vi "(SubVI)Waveform Editor.vi"() -> ()   [LabVIEW 2020]
uses:
  Libraries/Waveform Obj Class/Waveform Gen/Controls/repeat scale.ctl
  Libraries/Waveform Obj Class/Square Wave/Controls/Slope Type.ctl
  Libraries/Waveform Obj Class/Waveform Obj/Waveform Obj.lvclass
  Controls/(Ctrl)Waveform Editor_Update Listbox User Event.ctl
  Controls/(Ctrl)Waveform Editor_WF List.ctl
  Controls/(Ctrl)Waveform Editor_Update Graph User Event.ctl
  <vilib>/Utility/miscctls.llb/LVPointTypeDef.ctl
  Mode Event/Controls/(Ctrl)Mode Event_FGV Function.ctl
  Controls/(Ctrl)Waveform Editor_Update Sampling Rate Value.ctl
  Libraries/Haptic IC Class/Haptic IC/Haptic IC.lvclass/Haptic IC.ctl
  Libraries/Waveform Obj Class/Waveform Gen/Controls/waveform gen type.ctl
  Libraries/Waveform Obj Class/Sine Wave/Sine Wave.lvclass
  Libraries/Waveform Obj Class/Square Wave/Square Wave.lvclass
  Libraries/Waveform Obj Class/Square Wave/Square Wave.lvclass/Square Wave.ctl
  Libraries/Waveform Obj Class/Triangle Wave/Triangle Wave.lvclass
  Libraries/Waveform Obj Class/Sawtooth Wave/Sawtooth Wave.lvclass
  Libraries/Waveform Obj Class/Auto Track Wave/Auto Track Wave.lvclass
  Libraries/Waveform Obj Class/Auto Brake (Square) Wave/Auto Brake (Square) Wave.lvclass
  Libraries/Waveform Obj Class/Auto Brake (Sine) Wave/Auto Brake (Sine) Wave.lvclass
  Libraries/Waveform Obj Class/PWL_DW7802/PWL_DW7802.lvclass
  Libraries/Waveform Obj Class/Waveform Gen/Waveform Gen.lvclass/Waveform Gen.ctl
  Libraries/Waveform Obj Class/Waveform Obj/Waveform Obj.lvclass/Waveform Obj.ctl
  Libraries/Waveform Obj Class/Waveform Gen/Waveform Gen.lvclass
  Libraries/Waveform Obj Class/PWL/PWL.lvclass
  Libraries/Waveform Obj Class/PWL/PWL.lvclass/PWL.ctl
  Libraries/Waveform Obj Class/WAV File/WAV File.lvclass
  Libraries/Waveform Obj Class/Text File/Text File.lvclass
  Libraries/Haptic IC Class/Haptic IC/Controls/(Ctrl)Mode.ctl
  Mode Event/Controls/(Ctrl)Mode Event_Event Type.ctl
  Libraries/Waveform Obj Class/Square Wave/Accessors/Write slope length.vi
  Libraries/Waveform Obj Class/Square Wave/Accessors/Write slope type.vi
  Libraries/Waveform Obj Class/Waveform Gen/Accessors/Write frequency.vi
  Libraries/Waveform Obj Class/Waveform Gen/Accessors/Write scale.vi
  Libraries/Waveform Obj Class/Waveform Gen/Accessors/Write cycle.vi
  Libraries/Waveform Obj Class/Waveform Gen/Accessors/Write repeat type.vi
  Libraries/Waveform Obj Class/Waveform Obj/Accessors/Write sampling rate.vi
  Libraries/Waveform Obj Class/Waveform Obj/Accessors/Write voltage range.vi
  Libraries/Waveform Obj Class/Waveform Obj/Accessors/Write wait.vi
  9968c254-cfa1-4b75-a9b0-3c7b6300c374.vi
  Libraries/Waveform Obj Class/Waveform Obj/Accessors/Write name.vi
  Libraries/Waveform Obj Class/Square Wave/Accessors/Read slope length.vi
  Libraries/Waveform Obj Class/Square Wave/Accessors/Read slope type.vi
  Libraries/Waveform Obj Class/PWL/Accessors/Read previous pwl scale.vi
  Libraries/Waveform Obj Class/PWL/Accessors/Read waveform type.vi
  Libraries/Waveform Obj Class/Waveform Gen/Accessors/Read frequency.vi
  Libraries/Waveform Obj Class/Waveform Gen/Accessors/Read scale.vi
  Libraries/Waveform Obj Class/Waveform Gen/Accessors/Read cycle.vi
  Libraries/Waveform Obj Class/Waveform Gen/Accessors/Read repeat type.vi
  Libraries/Waveform Obj Class/Waveform Obj/Accessors/Read play mode.vi
  Libraries/Waveform Obj Class/PWL/Accessors/Write waveform type.vi
  Libraries/Waveform Obj Class/Waveform Obj/Accessors/Write play mode.vi
  Libraries/Waveform Obj Class/PWL/Accessors/Write previous pwl scale.vi
  073afacf-4daa-4c2b-8e37-4aa6efe5eb82.vi
  Libraries/Waveform Obj Class/Waveform Obj/Accessors/Read name.vi
  Libraries/Waveform Obj Class/Waveform Obj/Accessors/Read wait.vi
  Variables/(Var)System Variables.vi
  <vilib>/Comparison/Less/Less Functor/Less Functor.lvclass
  Libraries/Haptic IC Class/Haptic IC/Haptic IC.lvclass
panel:
  in  "WF Seq_PWL Points":u8(ring)=1 caption="PWL points" items=["1"=1, "2"=2, "3"=3, "4"=4, "5"=5, "6"=6, "7"=7]
  in  "WF Seq_Play Mode":u8(ring)
  in  "WF Seq_PWL_DW7802":T1(array[cluster])=[{"Shape"=0, "Ramp"=0, "Amplitude"=1.0, "Frequency"=100.0, "Cycle"=1.0}] {"Frequency" min=40.0 max=300.0 step=1.0; "Cycle" items=["0.5"=0.5, "1"=1.0, "1.5"=1.5, "2"=2.0, "2.5"=2.5, "3"=3.0, "3.5"=3.5, "4"=4.0, "4.5"=4.5, "5"=5.0, "5.5"=5.5, "6"=6.0, "6.5"=6.5, "7"=7.0, "7.5"=7.5, "8"=8.0, "8.5"=8.5, "9"=9.0, "9.5"=9.5, "10"=10.0, "10.5"=10.5, "11"=11.0, "11.5"=11.5, "12"=12.0, "12.5"=12.5, "13"=13.0, "13.5"=13.5, "14"=14.0, "14.5"=14.5, "15"=15.0, "15.5"=15.5, "16"=16.0, "16.5"=16.5, "17"=17.0, "17.5"=17.5, "18"=18.0, "18.5"=18.5, "19"=19.0, "19.5"=19.5, "20"=20.0, "20.5"=20.5, "21"=21.0, "21.5"=21.5, "22"=22.0, "22.5"=22.5, "23"=23.0, "23.5"=23.5, "24"=24.0, "24.5"=24.5, "25"=25.0, "25.5"=25.5, "26"=26.0, "26.5"=26.5, "27"=27.0, "27.5"=27.5, "28"=28.0, "28.5"=28.5, "29"=29.0, "29.5"=29.5, "30"=30.0, "30.5"=30.5, "31"=31.0, "31.5"=31.5, "32"=32.0, "32.5"=32.5, "33"=33.0, "33.5"=33.5, "34"=34.0, "34.5"=34.5, "35"=35.0, "35.5"=35.5, "36"=36.0, "36.5"=36.5, "37"=37.0, "37.5"=37.5, "38"=38.0, "38.5"=38.5, "39"=39.0, "39.5"=39.5, "40"=40.0, "40.5"=40.5, "41"=41.0, "41.5"=41.5, "42"=42.0, "42.5"=42.5, "43"=43.0, "43.5"=43.5, "44"=44.0, "44.5"=44.5, "45"=45.0, "45.5"=45.5, "46"=46.0, "46.5"=46.5, "47"=47.0, "47.5"=47.5, "48"=48.0, "48.5"=48.5, "49"=49.0, "49.5"=49.5, "50"=50.0, "50.5"=50.5, "51"=51.0, "51.5"=51.5, "52"=52.0, "52.5"=52.5, "53"=53.0, "53.5"=53.5, "54"=54.0, "54.5"=54.5, "55"=55.0, "55.5"=55.5, "56"=56.0, "56.5"=56.5, "57"=57.0, "57.5"=57.5, "58"=58.0, "58.5"=58.5, "59"=59.0, "59.5"=59.5, "60"=60.0, "60.5"=60.5, "61"=61.0, "61.5"=61.5, "62"=62.0, "62.5"=62.5, "63"=63.0, "63.5"=63.5, "64"=64.0, "64.5"=64.5, "65"=65.0, "65.5"=65.5, "66"=66.0, "66.5"=66.5, "67"=67.0, "67.5"=67.5, "68"=68.0, "68.5"=68.5, "69"=69.0, "69.5"=69.5, "70"=70.0, "70.5"=70.5, "71"=71.0, "71.5"=71.5, "72"=72.0, "72.5"=72.5, "73"=73.0, "73.5"=73.5, "74"=74.0, "74.5"=74.5, "75"=75.0, "75.5"=75.5, "76"=76.0, "76.5"=76.5, "77"=77.0, "77.5"=77.5, "78"=78.0, "78.5"=78.5, "79"=79.0, "79.5"=79.5, "80"=80.0, "80.5"=80.5, "81"=81.0, "81.5"=81.5, "82"=82.0, "82.5"=82.5, "83"=83.0, "83.5"=83.5, "84"=84.0, "84.5"=84.5, "85"=85.0, "85.5"=85.5, "86"=86.0, "86.5"=86.5, "87"=87.0, "87.5"=87.5, "88"=88.0, "88.5"=88.5, "89"=89.0, "89.5"=89.5, "90"=90.0, "90.5"=90.5, "91"=91.0, "91.5"=91.5, "92"=92.0, "92.5"=92.5, "93"=93.0, "93.5"=93.5, "94"=94.0, "94.5"=94.5, "95"=95.0, "95.5"=95.5, "96"=96.0, "96.5"=96.5, "97"=97.0, "97.5"=97.5, "98"=98.0, "98.5"=98.5, "99"=99.0, "99.5"=99.5, "100"=100.0, "100.5"=100.5, "101"=101.0, "101.5"=101.5, "102"=102.0, "102.5"=102.5, "103"=103.0, "103.5"=103.5, "104"=104.0, "104.5"=104.5, "105"=105.0, "105.5"=105.5, "106"=106.0, "106.5"=106.5, "107"=107.0, "107.5"=107.5, "108"=108.0, "108.5"=108.5, "109"=109.0, "109.5"=109.5, "110"=110.0, "110.5"=110.5, "111"=111.0, "111.5"=111.5, "112"=112.0, "112.5"=112.5, "113"=113.0, "113.5"=113.5, "114"=114.0, "114.5"=114.5, "115"=115.0, "115.5"=115.5, "116"=116.0, "116.5"=116.5, "117"=117.0, "117.5"=117.5, "118"=118.0, "118.5"=118.5, "119"=119.0, "119.5"=119.5, "120"=120.0, "120.5"=120.5, "121"=121.0, "121.5"=121.5, "122"=122.0, "122.5"=122.5, "123"=123.0, "123.5"=123.5, "124"=124.0, "124.5"=124.5, "125"=125.0, "125.5"=125.5, "126"=126.0, "126.5"=126.5, "127"=127.0, "127.5"=127.5]; "Amplitude" items=["0"=0.0, "10"=0.1, "20"=0.2, "30"=0.3, "40"=0.4, "50"=0.5, "60"=0.6, "70"=0.7, "80"=0.8, "90"=0.9, "100"=1.0]; "Ramp" items=["Step"=0, "Ramp (Lin.)"=2, "Ramp (Exp.)"=3]; "Shape" items=["Sine", "Square"]}
  in  "WF Seq_PWL Listbox":i32[](listbox)
  out "WF Gen_Auto Tracking Waring":string="Warning!\nThe center frequency of tracking range is out of range in the default ZXD Setting."
  in  "WF Seq_Wait":u8(ring) caption="Wait" items=["0us", "166us", "332us", "498us", "664us", "830us", "996us", "1162us", "1328us", "1494us", "1660us", "1826us", "1992us", "2158us", "2324us", "2490us"]
  in  "WF List_Mem Update":bool
  in  "WF List_RTP Stop":bool
  in  "WF List_RTP Start":bool
  in  "WF Seq_Voltage Range":dbl(ring) caption="VD Clamp" items=["0.00V"=0.0, "0.04V"=0.04, "0.08V"=0.08, "0.12V"=0.12, "0.16V"=0.16, "0.20V"=0.2, "0.24V"=0.24, "0.28V"=0.28, "0.32V"=0.32, "0.36V"=0.36, "0.40V"=0.4, "0.44V"=0.44, "0.48V"=0.48, "0.52V"=0.52, "0.56V"=0.56, "0.60V"=0.6, "0.64V"=0.64, "0.68V"=0.68, "0.72V"=0.72, "0.76V"=0.76, "0.80V"=0.8, "0.84V"=0.84, "0.88V"=0.88, "0.92V"=0.92, "0.96V"=0.96, "1.00V"=1.0, "1.04V"=1.04, "1.08V"=1.08, "1.12V"=1.12, "1.16V"=1.16, "1.20V"=1.2, "1.24V"=1.24, "1.28V"=1.28, "1.32V"=1.32, "1.36V"=1.36, "1.40V"=1.4, "1.44V"=1.44, "1.48V"=1.48, "1.52V"=1.52, "1.56V"=1.56, "1.60V"=1.6, "1.64V"=1.64, "1.68V"=1.68, "1.72V"=1.72, "1.76V"=1.76, "1.80V"=1.8, "1.84V"=1.84, "1.88V"=1.88, "1.92V"=1.92, "1.96V"=1.96, "2.00V"=2.0, "2.04V"=2.04, "2.08V"=2.08, "2.12V"=2.12, "2.16V"=2.16, "2.20V"=2.2, "2.24V"=2.24, "2.28V"=2.28, "2.32V"=2.32, "2.36V"=2.36, "2.40V"=2.4, "2.44V"=2.44, "2.48V"=2.48, "2.52V"=2.52, "2.56V"=2.56, "2.60V"=2.6, "2.64V"=2.64, "2.68V"=2.68, "2.72V"=2.72, "2.76V"=2.76, "2.80V"=2.8, "2.84V"=2.84, "2.88V"=2.88, "2.92V"=2.92, "2.96V"=2.96, "3.00V"=3.0, "3.04V"=3.04, "3.08V"=3.08, "3.12V"=3.12, "3.16V"=3.16, "3.20V"=3.2, "3.24V"=3.24, "3.28V"=3.28, "3.32V"=3.32, "3.36V"=3.36, "3.40V"=3.4, "3.44V"=3.44, "3.48V"=3.48, "3.52V"=3.52, "3.56V"=3.56, "3.60V"=3.6, "3.64V"=3.64, "3.68V"=3.68, "3.72V"=3.72, "3.76V"=3.76, "3.80V"=3.8, "3.84V"=3.84, "3.88V"=3.88, "3.92V"=3.92, "3.96V"=3.96, "4.00V"=4.0, "4.04V"=4.04, "4.08V"=4.08, "4.12V"=4.12, "4.16V"=4.16, "4.20V"=4.2, "4.24V"=4.24, "4.28V"=4.28, "4.32V"=4.32, "4.36V"=4.36, "4.40V"=4.4, "4.44V"=4.44, "4.48V"=4.48, "4.52V"=4.52, "4.56V"=4.56, "4.60V"=4.6, "4.64V"=4.64, "4.68V"=4.68, "4.72V"=4.72, "4.76V"=4.76, "4.80V"=4.8, "4.84V"=4.84, "4.88V"=4.88, "4.92V"=4.92, "4.96V"=4.96, "5.00V"=5.0, "5.04V"=5.04, "5.08V"=5.08, "5.12V"=5.12, "5.16V"=5.16, "5.20V"=5.2, "5.24V"=5.24, "5.28V"=5.28, "5.32V"=5.32, "5.36V"=5.36, "5.40V"=5.4, "5.44V"=5.44, "5.48V"=5.48, "5.52V"=5.52, "5.56V"=5.56, "5.60V"=5.6, "5.64V"=5.64, "5.68V"=5.68, "5.72V"=5.72, "5.76V"=5.76, "5.80V"=5.8, "5.84V"=5.84, "5.88V"=5.88, "5.92V"=5.92, "5.96V"=5.96, "6.00V"=6.0, "6.04V"=6.04, "6.08V"=6.08, "6.12V"=6.12, "6.16V"=6.16, "6.20V"=6.2, "6.24V"=6.24, "6.28V"=6.28, "6.32V"=6.32, "6.36V"=6.36, "6.40V"=6.4, "6.44V"=6.44, "6.48V"=6.48, "6.52V"=6.52, "6.56V"=6.56, "6.60V"=6.6, "6.64V"=6.64, "6.68V"=6.68, "6.72V"=6.72, "6.76V"=6.76, "6.80V"=6.8, "6.84V"=6.84, "6.88V"=6.88, "6.92V"=6.92, "6.96V"=6.96, "7.00V"=7.0, "7.04V"=7.04, "7.08V"=7.08, "7.12V"=7.12, "7.16V"=7.16, "7.20V"=7.2, "7.24V"=7.24, "7.28V"=7.28, "7.32V"=7.32, "7.36V"=7.36, "7.40V"=7.4, "7.44V"=7.44, "7.48V"=7.48, "7.52V"=7.52, "7.56V"=7.56, "7.60V"=7.6, "7.64V"=7.64, "7.68V"=7.68, "7.72V"=7.72, "7.76V"=7.76, "7.80V"=7.8, "7.84V"=7.84, "7.88V"=7.88, "7.92V"=7.92, "7.96V"=7.96, "8.00V"=8.0, "8.04V"=8.04, "8.08V"=8.08, "8.12V"=8.12, "8.16V"=8.16, "8.20V"=8.2, "8.24V"=8.24, "8.28V"=8.28, "8.32V"=8.32, "8.36V"=8.36, "8.40V"=8.4, "8.44V"=8.44, "8.48V"=8.48, "8.52V"=8.52, "8.56V"=8.56, "8.60V"=8.6, "8.64V"=8.64, "8.68V"=8.68, "8.72V"=8.72, "8.76V"=8.76, "8.80V"=8.8, "8.84V"=8.84, "8.88V"=8.88, "8.92V"=8.92, "8.96V"=8.96, "9.00V"=9.0, "9.04V"=9.04, "9.08V"=9.08, "9.12V"=9.12, "9.16V"=9.16, "9.20V"=9.2, "9.24V"=9.24, "9.28V"=9.28, "9.32V"=9.32, "9.36V"=9.36, "9.40V"=9.4, "9.44V"=9.44, "9.48V"=9.48, "9.52V"=9.52, "9.56V"=9.56, "9.60V"=9.6, "9.64V"=9.64, "9.68V"=9.68, "9.72V"=9.72, "9.76V"=9.76, "9.80V"=9.8, "9.84V"=9.84, "9.88V"=9.88, "9.92V"=9.92, "9.96V"=9.96, "10.00V"=10.0, "10.04V"=10.04, "10.08V"=10.08, "10.12V"=10.12, "10.16V"=10.16, "10.20V"=10.2]
  in  "WF List_Import":bool
  out "Graph_Cursor Y":dbl caption="Y :" format="Y : %#.3f"
  out "Graph_Cursor X":dbl caption="Cursor X :" format="X : %#_g"
  out "WF List_Total Bytes":i32 caption="Total :" format="%d Byte"
  out "WF Seq_Total Bytes":i32 caption="Total :" format="%d Byte"
  out "Graph":dbl[](graph)
  in  "WF List_Export":bool
  in  "WF List_Load File":bool
  in  "WF List_Save File":bool
  in  "WF List_Delete":bool
  in  "WF List_Rename":bool
  in  "WF List_Down":bool
  in  "WF List_Up":bool
  in  "WF List_View":bool
  in  "WF Seq_Change":bool
  in  "WF Seq_Add to List":bool
  in  "WF Seq_Load File":bool
  in  "WF Seq_Save File":bool
  in  "WF Seq_Delete":bool
  in  "WF Seq_Rename":bool
  in  "WF Seq_Down":bool
  in  "WF Seq_Up":bool
  in  "WF Seq_View":bool
  in  "WF Gen_Change":bool
  in  "WF Gen_Add to Seq":bool
  in  "WF List_Sampling Rate":u32(ring)=8000 caption="PWM" items=["24kHz"=24000, "48kHz"=48000, "96kHz"=96000, "12kHz"=12000]
  in  "WF Seq":i32[](listbox)
  in  "WF List":i32[](listbox)
  in  "WF Gen_Setting":T4={"Waveform Type"=0, "Freq."=160.0, "Scale"=1.0, "Cycle"=1.0, "Repeat Type"=enum."Normal", "Square_Slope Length"=25, "Square_Slope"=enum."Exp."} {"Scale" min=-1.0 max=1.0; "Waveform Type" items=["Sine", "Square", "Triangle", "Sawtooth"]}
  # "Waveform Editor"
  # "Cursor"
  # "Waveform Generate"
  # "Waveform Build"
  # "Waveform List"
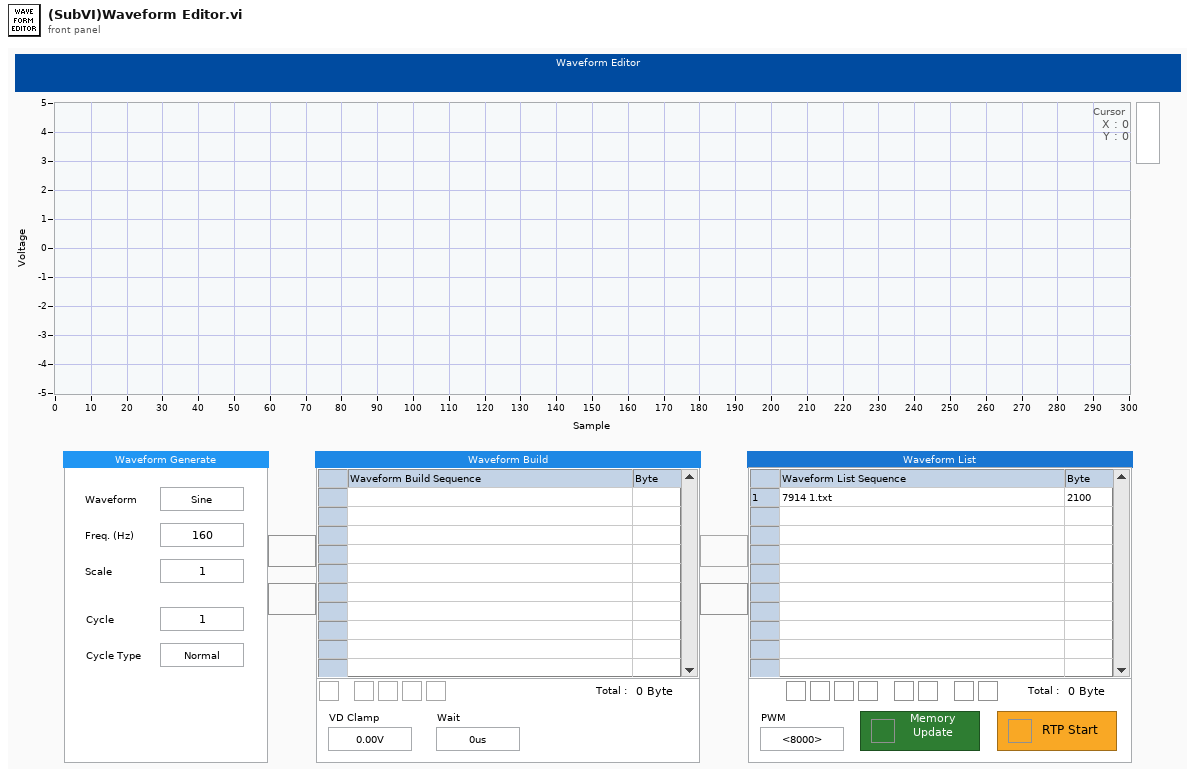
[diagram p1: front panel]
types:
  T1 = cluster{"Shape":u16, "Ramp":u16, "Amplitude":dbl, "Frequency":dbl, "Cycle":dbl}[]
  T2 = typedef "Waveform Gen.lvclass/repeat scale.ctl" = enum16{"Normal", "Lin. Up", "Lin. Down", "Exp. Up", "Exp. Down"}
  T3 = typedef "Square Wave.lvclass/Slope Type.ctl" = enum16{"None", "Lin.", "Exp."}
  T4 = cluster{"Waveform Type":u16, "Freq.":dbl, "Scale":dbl, "Cycle":dbl, "Repeat Type":T2, "Square_Slope Length":u32, "Square_Slope":T3}
  T5 = typedef "(Ctrl)Mode Event_FGV Function.ctl" = enum16{"Init", "Get Event Ref", "Gen Event", "Destroy"}
  T6 = typedef "LVPointTypeDef.ctl" = cluster{"Horizontal":i16, "Vertical":i16}
  T7 = typedef "(Ctrl)Waveform Editor_Update Graph User Event.ctl" = enum16{"WF Gen", "WF Seq", "Latest"}
  T8 = typedef "(Ctrl)Waveform Editor_Update Listbox User Event.ctl" = enum16{"WF Seq", "WF List"}
  T9 = typedef "(Ctrl)Waveform Editor_WF List.ctl" = cluster{"Name":string, "WF Seq":refnum<class "Waveform Obj.lvclass">[]}
  T10 = typedef "(Ctrl)Waveform Editor_Update Sampling Rate Value.ctl" = enum16{"Init", "Update"}
  T11 = typedef "Haptic IC.lvclass/(Ctrl)IC Type.ctl" = enum8{"DW7800", "DW7802", "DW7912", "DW7914"}
  T12 = typedef "Waveform Gen.lvclass/waveform gen type.ctl" = enum16{"Sine", "Square", "Triangle", "Sawtooth", "Auto Track", "Auto Brake (Square)", "Auto Brake (Sine)", "PWL"}
  T13 = typedef "LVStringsAndValuesArrayTypeDef_DBL.ctl" = cluster{"String":string, "Value":dbl}[]
  T14 = typedef "LVStringsAndValuesArrayTypeDef_U32.ctl" = cluster{"String":string, "Value":u32}[]
  T15 = typedef "LVStringsAndValuesArrayTypeDef_U8.ctl" = cluster{"String":string, "Value":u8}[]
  T16 = enum16{"open", "replace", "create", "open or create", "replace or create", "replace or create with confirmation"}
  T17 = enum8{"Enabled", "Disabled", "Disabled and Grayed Out"}
  T18 = typedef "(Ctrl)Waveform Editor_Update Graph User Event.ctl" = enum16{"WF Gen", "WF Seq", "WF List", "Latest"}
  T19 = typedef "(Ctrl)Mode.ctl" = enum16{"RTP", "Memory"}
  T20 = typedef "(Ctrl)Mode Event_Event Type.ctl" = enum16{"RTP Play", "RTP Stop", "Scope Start", "Scope Stop"}
  T21 = typedef "LVRowAndColumnTypeDef.ctl" = cluster{"Row":i32, "Column":i32}
  T22 = typedef "LVPoint32TypeDef.ctl" = cluster{"Horizontal":i32, "Vertical":i32}
  T23 = cluster{"Shape":u16, "Ramp":u16, "Amplitude":dbl, "Frequency":dbl, "Cycle":dbl}
  T24 = cluster{"Accessors:waveform type":T12, "Accessors:repeat type":T2, "Accessors:scale":dbl, "Accessors:frequency":dbl, "Accessors:cycle":dbl}
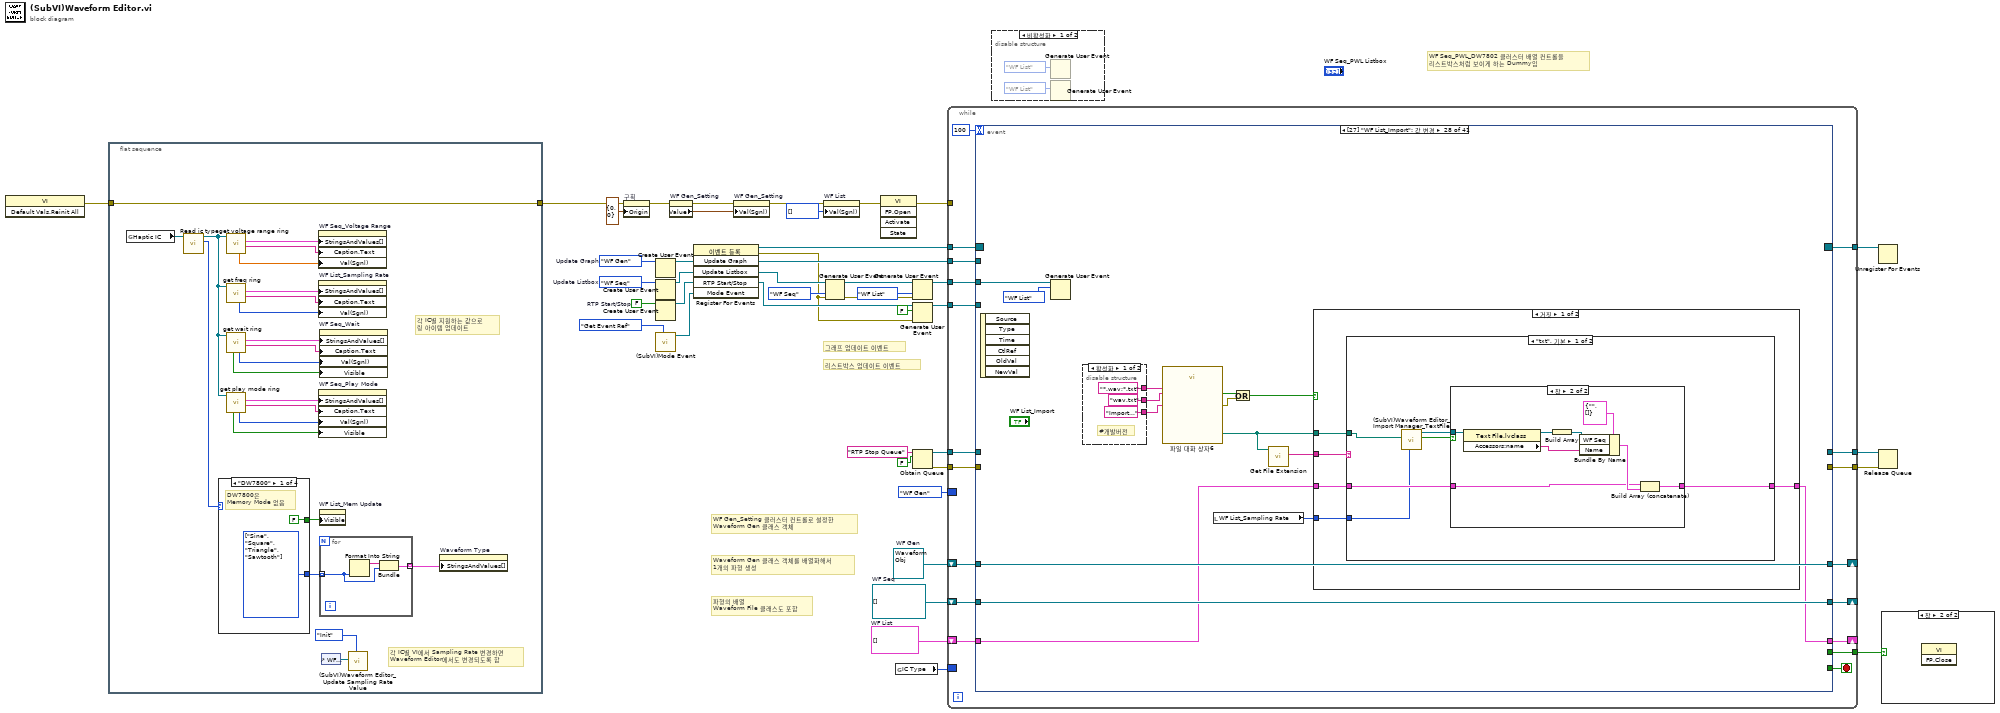
[diagram p0: block diagram]
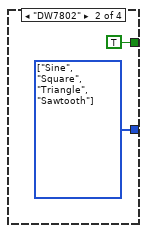
[diagram p3: hidden frame]
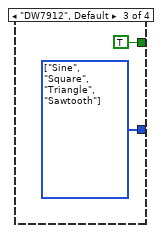
[diagram p4: hidden frame]
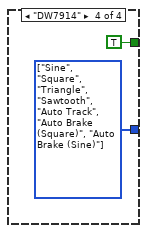
[diagram p5: hidden frame]
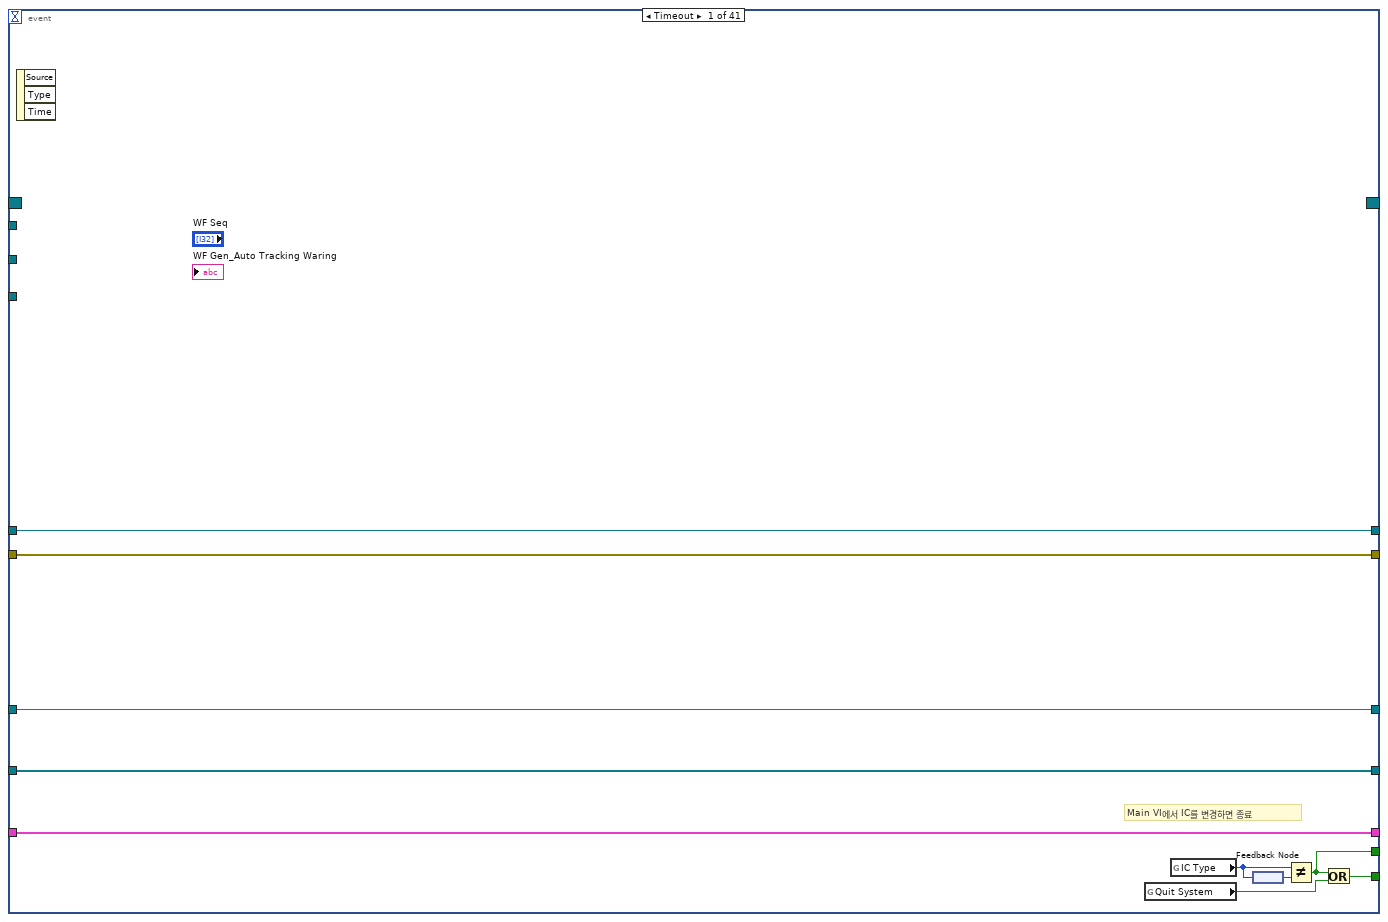
[diagram p7: hidden frame]
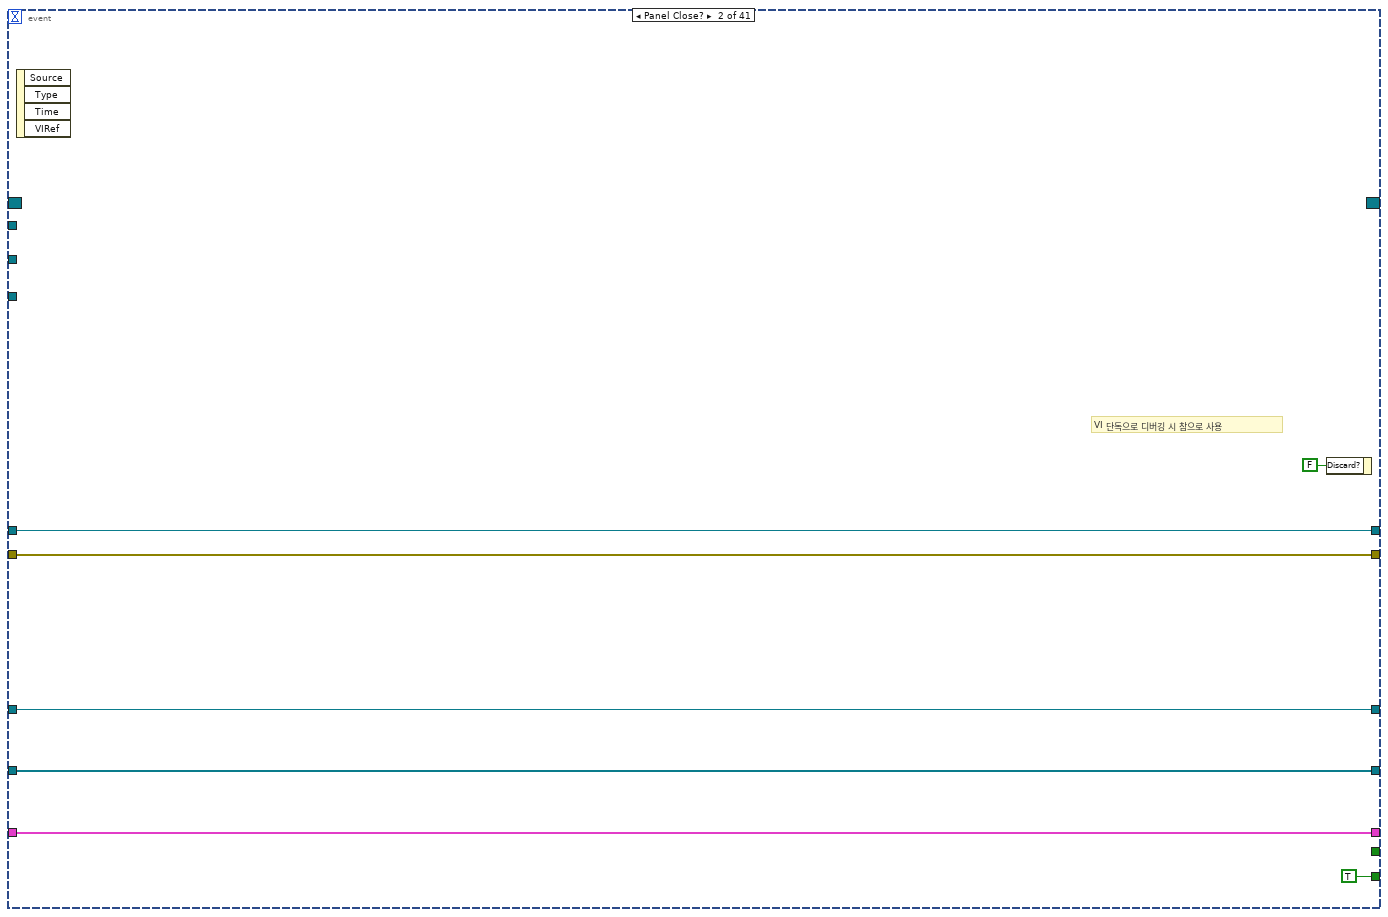
[diagram p8: hidden frame]
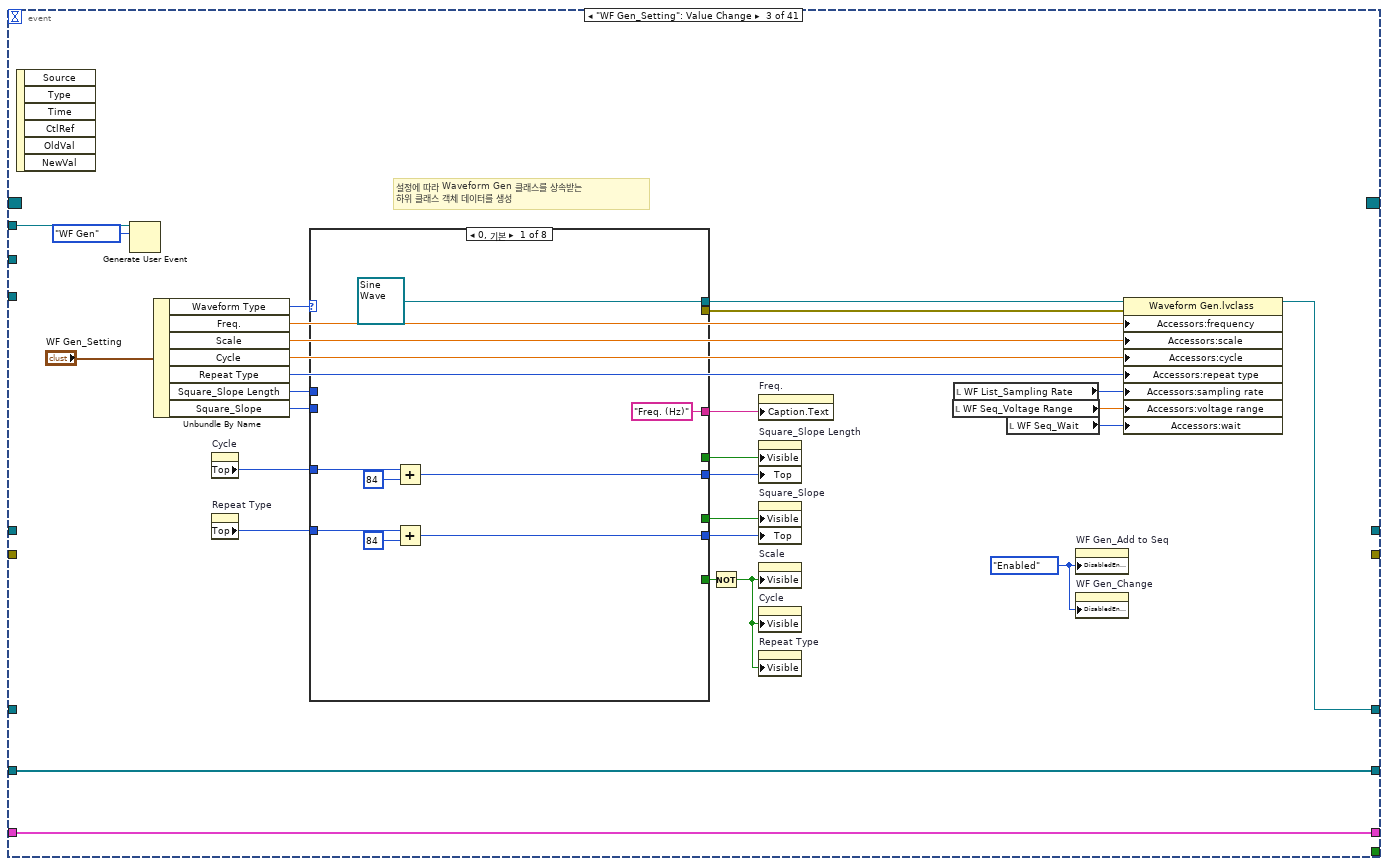
[diagram p9: hidden frame]
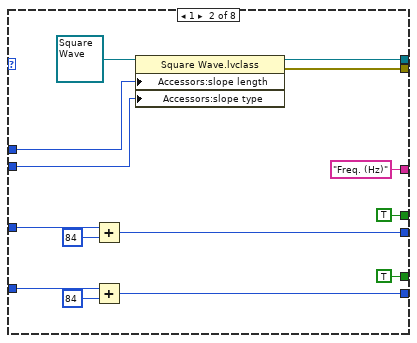
[diagram p10: hidden frame]
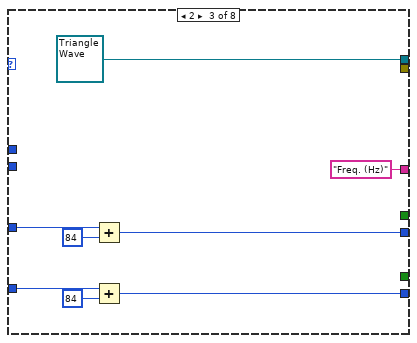
[diagram p11: hidden frame]
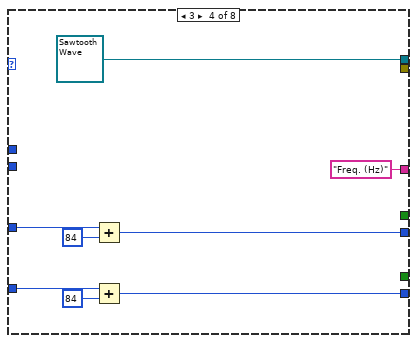
[diagram p12: hidden frame]
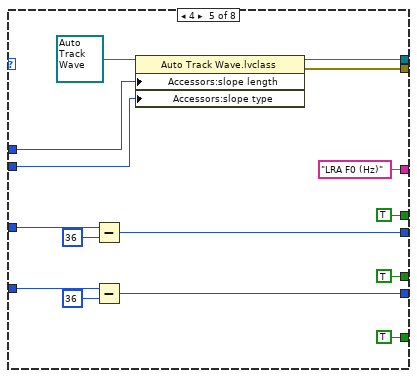
[diagram p13: hidden frame]
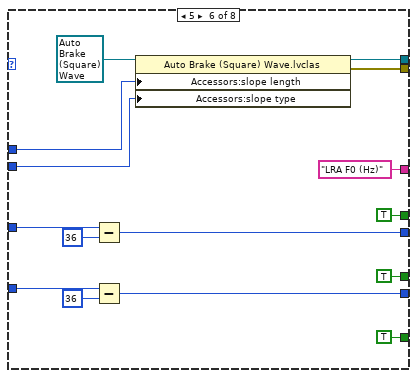
[diagram p14: hidden frame]
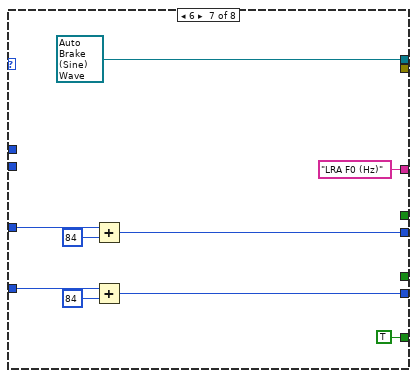
[diagram p15: hidden frame]
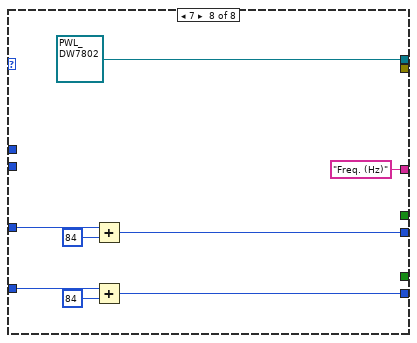
[diagram p16: hidden frame]
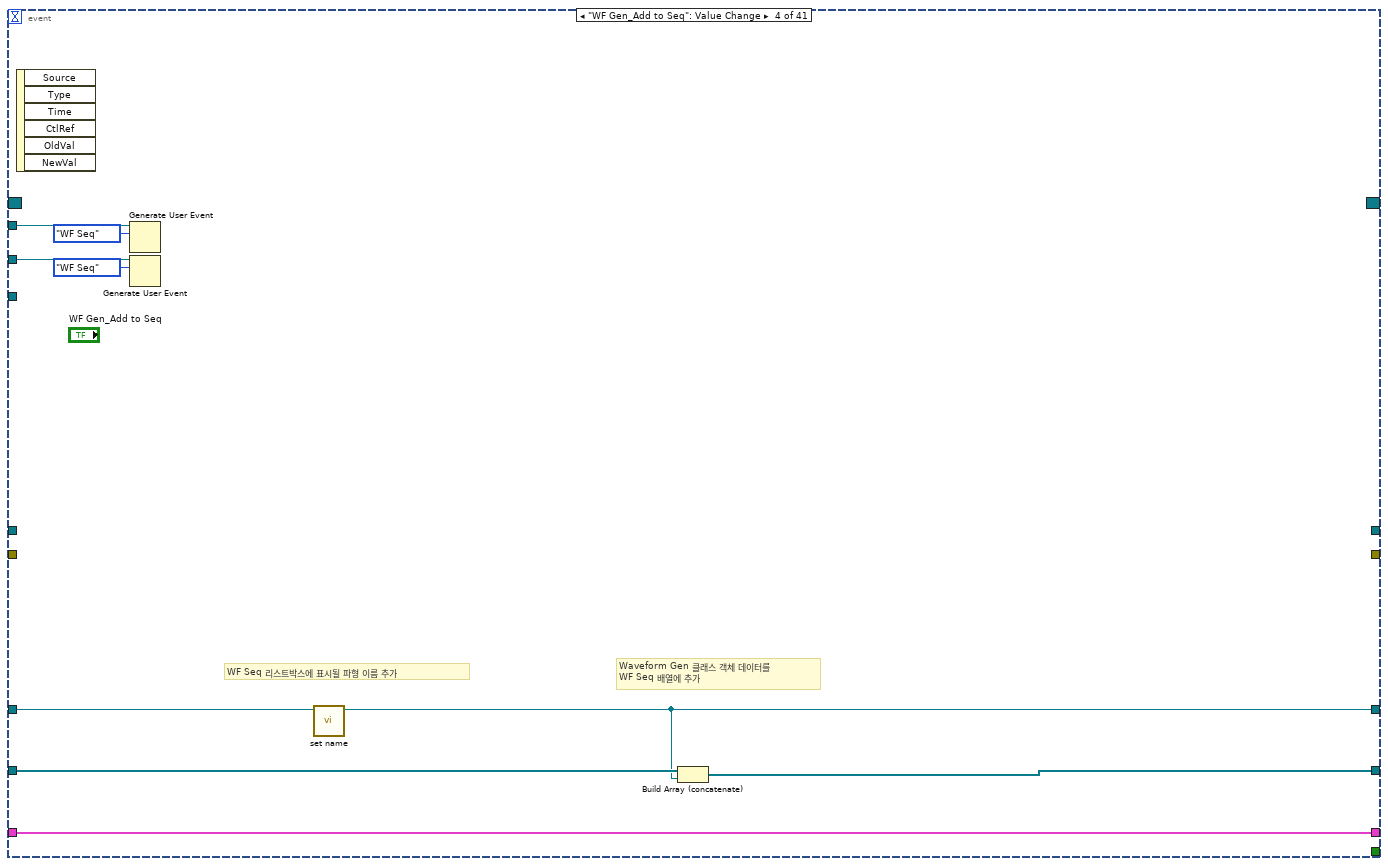
[diagram p17: hidden frame]
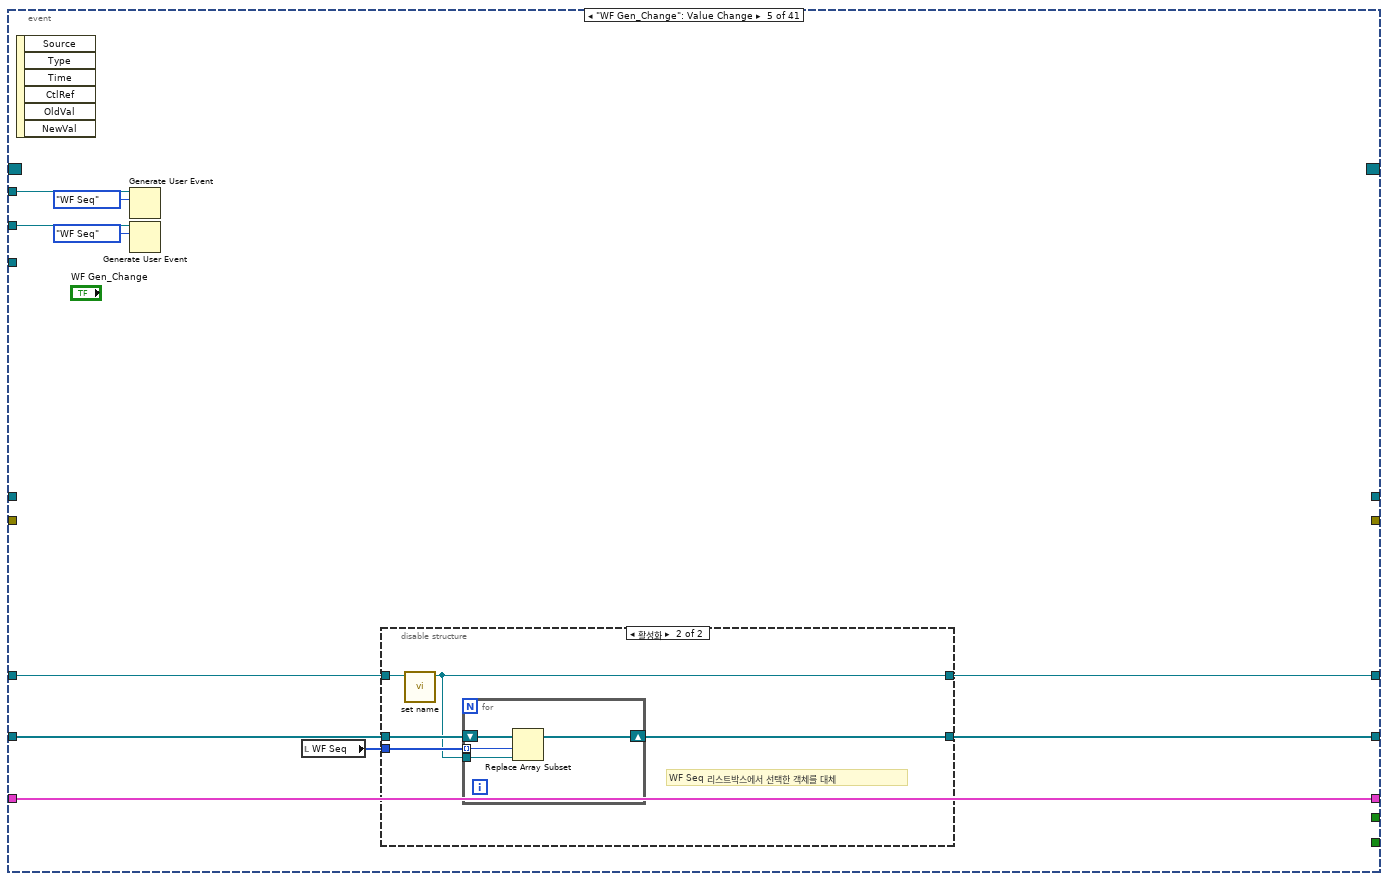
[diagram p18: hidden frame]
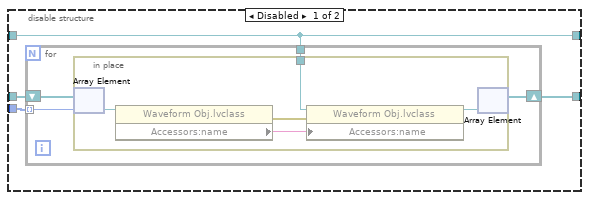
[diagram p19: hidden frame]
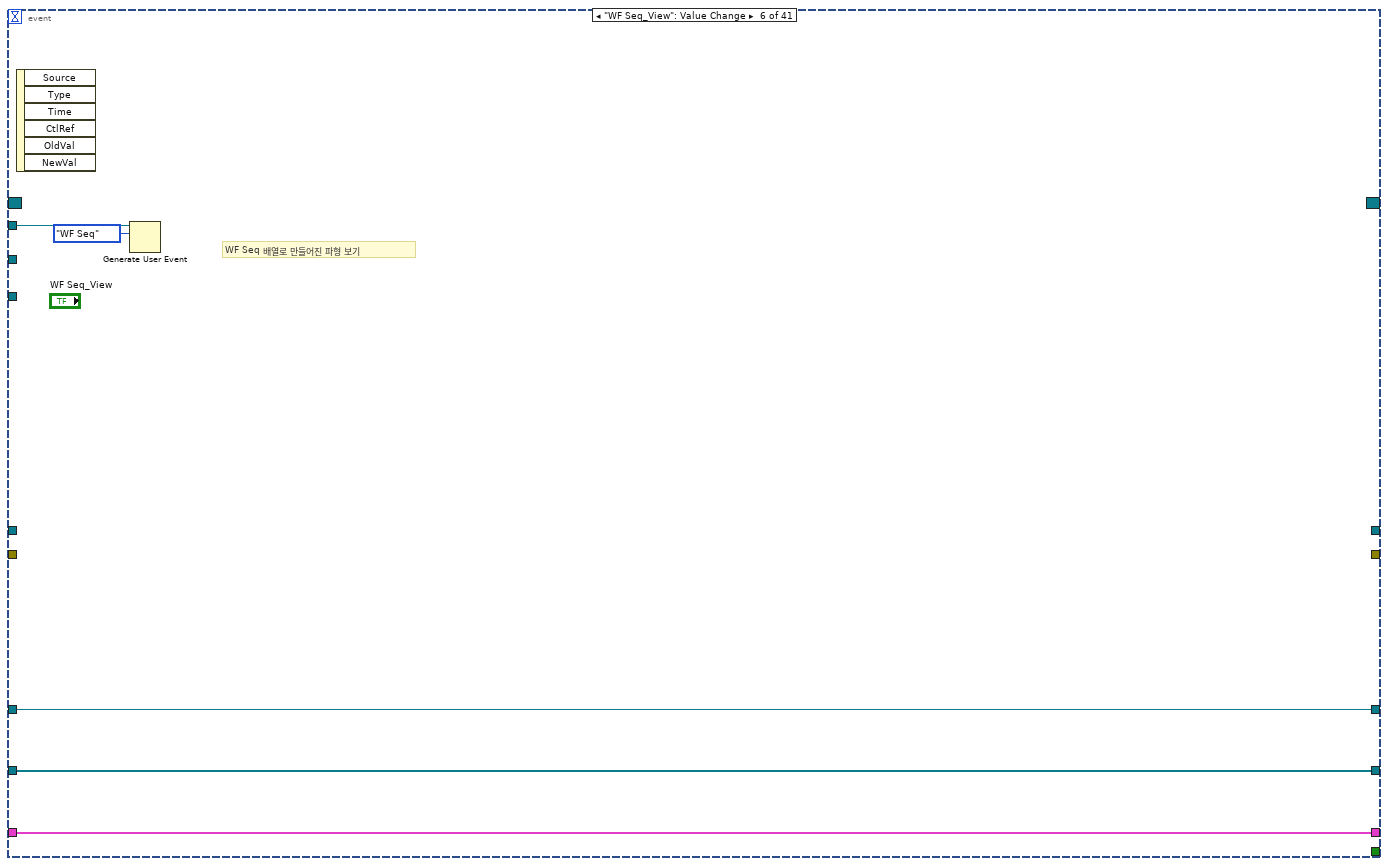
[diagram p20: hidden frame]
diagram:
  w14 = FALSE  # RTP Start/Stop
  w21 = T9[] []  # WF List
  w33 = (Ctrl)Waveform_Editor_Update_Listbox_User_Event."WF Seq"  # Update Listbox
  w36 = (Ctrl)Waveform_Editor_Update_Graph_User_Event."WF Gen"  # Update Graph
  w39 = refnum<class "Waveform Obj.lvclass"> refnum  # WF Gen
  w40 = refnum<class "Waveform Obj.lvclass">[] []  # WF Seq
  # "WF Seq_PWL_DW7802 클러스터 배열 컨트롤을\n리스트박스처럼 보이게 하는 Dummy임"
  # "리스트박스 업데이트 이벤트"
  # "그래프 업데이트 이벤트"
  # "파형의 배열\nWaveform File 클래스도 포함"
  # "Waveform Gen 클래스 객체를 배열화해서\n1개의 파형 생성"
  # "WF Gen_Setting 클러스터 컨트롤로 설정한\nWaveform Gen 클래스 객체"
  n1 = invoke class="VI" method="Default Vals.Reinit All"() -> (error out=w8:errorcluster)  [unwired: 3 in, 2 out]
  n2 = flat-sequence {
    tunnel: w8 -> [w56]
    tunnel: [w56] -> w6
    frame #0 {
      # "각 IC별 지원하는 값으로\n링 아이템 업데이트"
      # "각 IC별 VI에서 Sampling Rate 변경하면\nWaveform Editor에서도 변경되도록 함"
      n3 = global read "(Var)System Variables.vi" "Haptic IC"() -> (w59:refnum<class "Haptic IC.lvclass">)
      n4 = call "Read ic type.vi"("Haptic IC 입력"=w59) -> ("ic type"=w58:T11, "Haptic IC 출력"=w41:refnum<class "Haptic IC.lvclass">)  [unwired: 8 in, 1 out]
      n5 = case shown="\"DW7800\"" w58 {
        tunnel: [FALSE TRUE TRUE TRUE] -> w57
        tunnel: [w67 w69 w71 w73] -> w49
        frame "DW7800" {
          w67 = T12[] [enum."Sine", enum."Square", enum."Triangle", enum."Sawtooth"] items=["Sine", "Square", "Triangle", "Sawtooth", "Auto Track", "Auto Brake (Square)", "Auto Brake (Sine)", "PWL"] ("배열")
          # "DW7800은 \nMemory Mode 없음"
        }
        frame "DW7802" {
          w69 = T12[] [enum."Sine", enum."Square", enum."Triangle", enum."Sawtooth"] items=["Sine", "Square", "Triangle", "Sawtooth", "Auto Track", "Auto Brake (Square)", "Auto Brake (Sine)", "PWL"] ("배열")
        }
        frame "DW7912", Default {
          w71 = T12[] [enum."Sine", enum."Square", enum."Triangle", enum."Sawtooth"] items=["Sine", "Square", "Triangle", "Sawtooth", "Auto Track", "Auto Brake (Square)", "Auto Brake (Sine)", "PWL"] ("배열")
        }
        frame "DW7914" {
          w73 = T12[] [enum."Sine", enum."Square", enum."Triangle", enum."Sawtooth", enum."Auto Track", enum."Auto Brake (Square)", enum."Auto Brake (Sine)"] items=["Sine", "Square", "Triangle", "Sawtooth", "Auto Track", "Auto Brake (Square)", "Auto Brake (Sine)", "PWL"] ("배열")
        }
      }
      n6 = call-dynamic "get voltage range ring.vi"("Haptic IC 입력"=w41) -> ("caption"=w63:string, "strings & values"=w61:T13, "read value"=w51:dbl)  [unwired: 6 in, 2 out]
      n7 = call-dynamic "get freq ring.vi"("Haptic IC 입력"=w41) -> ("caption"=w62:string, "strings & values"=w60:T14, "read value"=w50:u32)  [unwired: 6 in, 2 out]
      n8 = call-dynamic "get wait ring.vi"("Haptic IC 입력"=w41) -> ("caption"=w54:string, "strings & values"=w55:T15, "default value"=w53:u8, "using"=w52:bool)  [unwired: 5 in, 2 out]
      n9 = call-dynamic "get play mode ring.vi"("Haptic IC 입력"=w41) -> ("caption"=w44:string, "strings & values"=w43:T15, "default value"=w45:u8, "using"=w42:bool)  [unwired: 5 in, 2 out]
      n10 = property on="WF Seq_Voltage Range" class="Ring (엄격한)"("StringsAndValues[]"=w61, "Caption.Text"=w63, "Val(Sgnl)"=w51) -> ()  [unwired: 2 in, 2 out]
      n11 = property on="WF List_Sampling Rate" class="Ring (엄격한)"("StringsAndValues[]"=w60, "Caption.Text"=w62, "Val(Sgnl)"=w50) -> ()  [unwired: 2 in, 2 out]
      n12 = property on="WF Seq_Play Mode" class="Ring (엄격한)"("StringsAndValues[]"=w43, "Caption.Text"=w44, "Val(Sgnl)"=w45, "Visible"=w42) -> ()  [unwired: 2 in, 2 out]
      n13 = property on="WF Seq_Wait" class="Ring (엄격한)"("StringsAndValues[]"=w55, "Caption.Text"=w54, "Val(Sgnl)"=w53, "Visible"=w52) -> ()  [unwired: 2 in, 2 out]
      n14 = property on="WF List_Mem Update" class="Bool"("Visible"=w57) -> ()  [unwired: 2 in, 2 out]
      n15 = for {
        tunnel: w49 -> [w65] mode=indexing
        tunnel: [w64] -> w48 mode=indexing
        n16 = Format Into String(w65) -> (resulting string=w66:string)  [unwired: 3 in, 1 out]
        n17 = Bundle(w66, "Waveform Type"=w65) -> (w64:cluster{string, "Waveform Type":T12})  [unwired: 1 in]
      }
      n18 = control-ref of="WF List_Sampling Rate"() -> (w47:refnum<vi>)
      n19 = call "(SubVI)Waveform Editor_Update Sampling Rate Value.vi"("Action"=(Ctrl)Waveform_Editor_Update_Sampling_Rate_Value."Init", "Sampling Rate Ref"=w47) -> ()  [unwired: 9 in, 1 out]
      n20 = property on="Waveform Type" class="Ring (엄격한)"("StringsAndValues[]"=w48) -> ()  [unwired: 2 in, 2 out]
    }
  }
  n21 = property on="구획" class="Pane"(error in=w6, "Origin"=T6 {"Horizontal"=0, "Vertical"=0} ("원점")) -> (error out=w30:errorcluster)  [unwired: 1 in, 1 out]
  n22 = Create User Event(user event datatype=w36) -> (user event=w34:refnum<user-event>)  [unwired: 1 in, 1 out]
  n23 = Create User Event(user event datatype=w33) -> (user event=w32:refnum<user-event>)  [unwired: 1 in, 1 out]
  n24 = Create User Event(user event datatype=w14) -> (user event=w13:refnum<user-event>)  [unwired: 1 in, 1 out]
  n25 = call "(SubVI)Mode Event.vi"("Function (Gen)"=(Ctrl)Mode_Event_FGV_Function."Get Event Ref" ("Function")) -> ("Mode Event"=w1:refnum<user-event>)  [unwired: 9 in, 1 out]
  n26 = property on="WF Gen_Setting" class="Clust (엄격한)"(error in=w30) -> (error out=w37:errorcluster, "Value"=w38:T4)  [unwired: 1 in, 1 out]
  n27 = register-events(w34, w32, w13, w1) -> (reference out=w35:refnum<event-registration>, error out=w10:errorcluster)  [unwired: 2 in]
  n28 = property on="WF Gen_Setting" class="Clust (엄격한)"(error in=w37, "Val(Sgnl)"=w38) -> (error out=w24:errorcluster)  [unwired: 1 in, 1 out]
  n29 = property on="WF List" class="MCListbox (엄격한)"(error in=w24, "Val(Sgnl)"=i32[] [] ("값(신호)")) -> (error out=w7:errorcluster)  [unwired: 1 in, 1 out]
  n30 = Generate User Event(user event=w32, event data cluster=(Ctrl)Waveform_Editor_Update_Listbox_User_Event."WF Seq" ("이벤트 데이터"), error in=w10) -> (user event out=w26:refnum<user-event>, error out=w25:errorcluster)  [unwired: 1 in]
  n31 = invoke class="VI" method="FP.Open"(error in=w7) -> (error out=w5:errorcluster)  [unwired: 4 in, 4 out]
  n32 = global read "(Var)System Variables.vi" "IC Type"() -> (w4:T11)
  n33 = Generate User Event(user event=w26, event data cluster=(Ctrl)Waveform_Editor_Update_Listbox_User_Event."WF List" ("이벤트 데이터"), error in=w25) -> (user event out=w27:refnum<user-event>)  [unwired: 1 in, 1 out]
  n34 = Generate User Event(user event=w13, event data cluster=FALSE ("이벤트 데이터"), error in=w10) -> (user event out=w12:refnum<user-event>)  [unwired: 1 in, 1 out]
  n35 = Obtain Queue(name (unnamed)="RTP Stop Queue" ("이름(이름없음)"), element data type=FALSE) -> (queue out=w18:refnum<queue>, error out=w17:errorcluster)  [unwired: 3 in, 1 out]
  n36 = while {
    shift-right: [w89] -> _
    shift-left: w40 -> [w90]
    shift-right: [w88] -> _
    shift-left: w39 -> [w87]
    tunnel: w35 -> [w86]
    tunnel: w34 -> [w85]
    tunnel: w27 -> [w84]
    shift-right: [w82] -> _
    shift-left: w21 -> [w83]
    tunnel: [w81] -> w29
    border: (Ctrl)Waveform_Editor_Update_Graph_User_Event."WF Gen" ("Update Graph") -> [_]
    tunnel: w18 -> [w80]
    tunnel: w17 -> [w79]
    tunnel: [w78] -> w16
    tunnel: [w77] -> w15
    tunnel: w12 -> [w76]
    tunnel: w5 -> [_]
    border: w4 -> [_]
    tunnel: [w75] -> w3
    stop <- w91 stop-if-true
    n37 = event shown="[27] \"WF List_Import\": 값 변경" {
      selector: w86 -> [_ _ _ _ _ _ _ _ _ _ _ _ _ _ _ _ _ _ _ _ _ _ _ _ _ _ _ _ _ _ _ _ _ _ _ _ _ _ _ _ _]
      dyn-events: [_ _ _ _ _ _ _ _ _ _ _ _ _ _ _ _ _ _ _ _ _ _ _ _ _ _ _ _ _ _ _ _ _ _ _ _ _ _ _ _ _] -> w81
      timeout: 100 -> [_ _ _ _ _ _ _ _ _ _ _ _ _ _ _ _ _ _ _ _ _ _ _ _ _ _ _ _ _ _ _ _ _ _ _ _ _ _ _ _ _]
      tunnel: [w94 TRUE _ _ _ _ _ _ _ _ _ _ _ _ _ _ _ _ _ _ _ _ _ _ _ _ _ _ _ _ _ _ _ _ _ _ _ _ _ _ _] -> w91
      tunnel: w90 -> [w102 w108 w137 w231 w241 w268 w276 w299 w330 w338 w351 w358 w377 w418 w476 w482 w517 _ w558 w563 w606 w621 w626 w648 w681 w684 w696 w719 w770 w775 w794 w835 w950 w971 w994 w1012 w1021 w1035 w1054 w1113 w1118]
      tunnel: [w102 w108 w137 w230 w240 w268 w275 w305 w330 w334 w349 w358 w376 w418 w473 w481 w517 w536 w558 w563 w606 w621 w626 w648 w681 w684 w696 w719 w770 w775 w794 w834 w947 w971 w994 w1012 w1021 w1035 w1054 w1113 w1118] -> w89
      tunnel: [w101 w107 w121 w229 w232 w267 w278 w306 w329 w339 w352 w365 w388 w421 w474 w484 w516 w539 w561 w570 w605 w620 w631 w657 w680 w690 w701 w718 w769 w780 w803 w842 w948 w970 w993 w1011 w1020 w1025 w1056 w1112 w1117] -> w88
      tunnel: w87 -> [w101 w107 _ w223 w238 w267 w278 w306 w329 w339 w352 w365 w388 w421 w475 w484 w516 w539 w561 w570 w605 w620 w631 w657 w680 w690 w701 w718 w769 w780 w803 w842 w949 w970 w993 w1011 w1020 w1036 w1056 w1112 w1117]
      tunnel: w85 -> [_ _ w123 w226 w235 w266 w271 w295 _ _ w346 _ w380 _ w471 w485 _ w534 _ _ _ w619 _ _ _ _ _ _ _ _ w796 w833 w945 _ _ _ _ _ _ _ _]
      tunnel: w84 -> [_ _ _ w225 w234 _ w270 w294 _ w332 w345 _ w379 _ _ w483 _ _ w554 w568 _ _ w624 w646 _ w685 w694 w711 _ _ w795 w832 w944 _ _ _ w1014 _ _ _ w1114]
      tunnel: w83 -> [w100 w105 w120 w224 w233 w264 w269 w293 w323 w331 w343 w359 w378 w417 w470 w487 w515 w538 w560 w567 w591 w618 w628 w650 w674 w683 w698 w710 w768 w773 w791 w831 w939 w968 w990 w1010 w1019 w1031 w1053 w1108 w1116]
      tunnel: [w100 w105 w120 w224 w233 w264 w269 w293 w323 w331 w343 w359 w378 w417 w470 w487 w515 w538 w559 w565 w591 w618 w627 w649 w674 w682 w697 w709 w768 w773 w792 w830 w938 w968 w990 w1010 w1019 w1031 w1053 w1108 w1116] -> w82
      tunnel: w80 -> [w99 w104 _ _ _ _ _ _ _ _ _ _ _ _ _ _ _ _ _ _ _ _ _ _ _ _ _ _ _ _ _ _ _ _ _ w1009 _ _ _ _ _]
      tunnel: w79 -> [w98 w103 _ _ _ _ _ _ _ _ _ _ _ _ _ _ _ _ _ _ _ _ _ _ _ _ _ _ _ _ _ _ _ _ _ w1008 _ _ _ _ _]
      tunnel: [w99 w104 _ _ _ _ _ _ _ _ _ _ _ _ _ _ _ _ _ _ _ _ _ _ _ _ _ _ _ _ _ _ _ _ _ _ _ _ _ _ _] -> w78
      tunnel: [w98 w103 _ _ _ _ _ _ _ _ _ _ _ _ _ _ _ _ _ _ _ _ _ _ _ _ _ _ _ _ _ _ _ _ _ _ _ _ _ _ _] -> w77
      tunnel: w76 -> [_ _ _ _ _ _ _ _ _ _ _ _ _ _ _ _ _ _ _ _ _ _ _ _ _ _ _ _ _ _ _ _ _ _ w974 _ _ _ _ _ _]
      tunnel: [w93 _ _ _ _ _ _ _ _ _ _ _ _ _ _ _ _ _ _ _ _ _ _ _ _ _ _ _ _ _ _ _ _ _ _ _ _ _ _ _ _] -> w75
      event Timeout {
        # "Main VI에서 IC를 변경하면 종료"
        n38 = event-data() -> ()  [unwired: 1 in, 3 out]
        n39 = global read "(Var)System Variables.vi" "Quit System"() -> (w95:bool)
        n40 = global read "(Var)System Variables.vi" "IC Type"() -> (w97:T11)
        n41 = feedback-in #1(w97) -> ()
        n42 = feedback #1() -> (w96:T11)
        n43 = Not Equal?(x=w97, y=w96) -> (x != y?=w93:bool)
        n44 = Or(x=w93, y=w95) -> (x .or. y?=w94:bool)
      }
      event Panel Close? {
        # "VI 단독으로 디버깅 시 참으로 사용"
        n45 = event-data() -> ()  [unwired: 1 in, 4 out]
        n46 = event-data("Discard?"=FALSE ("버림?")) -> ()  [unwired: 1 in, 1 out]
      }
      event "WF Gen_Setting": Value Change {
        w110 = T17."Enabled" ("비활성화")
        # "설정에 따라 Waveform Gen 클래스를 상속받는\n하위 클래스 객체 데이터를 생성"
        n47 = event-data() -> ()  [unwired: 1 in, 6 out]
        n48 = Generate User Event(user event=w123, event data cluster=(Ctrl)Waveform_Editor_Update_Graph_User_Event."WF Gen" ("이벤트 데이터")) -> ()  [unwired: 2 in, 2 out]
        n49 = Unbundle By Name("WF Gen_Setting") -> ("Waveform Type"=w135:u16, "Freq."=w132:dbl, "Scale"=w131:dbl, "Cycle"=w130:dbl, "Repeat Type"=w129:T2, "Square_Slope Length"=w127:u32, "Square_Slope"=w126:T3)
        n50 = property on="Cycle" class="DigNum (엄격한)"() -> ("Top"=w112:i32)  [unwired: 2 in, 2 out]
        n51 = property on="Repeat Type" class="Enum (엄격한)"() -> ("Top"=w111:i32)  [unwired: 2 in, 2 out]
        n52 = case shown="0, 기본" w135 {
          tunnel: [refnum<class "Sine Wave.lvclass"> refnum ("Sine Wave.lvclass") w158 refnum<class "Triangle Wave.lvclass"> refnum ("Triangle Wave.lvclass") refnum<class "Sawtooth Wave.lvclass"> refnum ("Sawtooth Wave.lvclass") w183 w198 refnum<class "Auto Brake (Sine) Wave.lvclass"> refnum ("Auto Brake (Sine) Wave.lvclass") refnum<class "PWL_DW7802.lvclass"> refnum ("PWL_DW7802.lvclass")] -> w134
          tunnel: [_ w157 _ _ w182 w197 _ _] -> w133
          tunnel: w127 -> [_ w156 _ _ w189 w204 _ _]
          tunnel: w126 -> [_ w155 _ _ w188 w203 _ _]
          tunnel: [_ TRUE _ _ TRUE TRUE _ _] -> w125
          tunnel: [_ TRUE _ _ TRUE TRUE _ _] -> w124
          tunnel: ["Freq. (Hz)" ("캡션.텍스트") "Freq. (Hz)" ("캡션.텍스트") "Freq. (Hz)" ("캡션.텍스트") "Freq. (Hz)" ("캡션.텍스트") "LRA F0 (Hz)" ("캡션.텍스트") "LRA F0 (Hz)" ("캡션.텍스트") "LRA F0 (Hz)" ("캡션.텍스트") "Freq. (Hz)" ("캡션.텍스트")] -> w117
          tunnel: [w141 w147 w161 w169 w177 w192 w208 w218] -> w116
          tunnel: [w138 w146 w160 w168 w176 w191 w207 w215] -> w115
          tunnel: [_ _ _ _ TRUE ("보이기") TRUE ("보이기") TRUE ("보이기") _] -> w114
          tunnel: w112 -> [w143 w149 w163 w171 w179 w194 w210 w220]
          tunnel: w111 -> [w139 w148 w162 w170 w178 w193 w209 w216]
          frame 0, Default {
            n53 = Add(x=w143, y=84) -> (x+y=w141:i32)
            n54 = Add(x=w139, y=84) -> (x+y=w138:i32)
          }
          frame 1 {
            n55 = Add(x=w149, y=84) -> (x+y=w147:i32)
            n56 = Add(x=w148, y=84) -> (x+y=w146:i32)
            n57 = property class="Square Wave.lvclass"(reference=refnum<class "Square Wave.lvclass"> refnum ("Square Wave.lvclass"), "Accessors:slope length"=w156, "Accessors:slope type"=w155) -> (reference out=w158:refnum<class "Square Wave.lvclass">, error out=w157:errorcluster)  [unwired: 1 in]
          }
          frame 2 {
            n58 = Add(x=w163, y=84) -> (x+y=w161:i32)
            n59 = Add(x=w162, y=84) -> (x+y=w160:i32)
          }
          frame 3 {
            n60 = Add(x=w171, y=84) -> (x+y=w169:i32)
            n61 = Add(x=w170, y=84) -> (x+y=w168:i32)
          }
          frame 4 {
            n62 = Subtract(x=w179, y=36) -> (x-y=w177:i32)
            n63 = Subtract(x=w178, y=36) -> (x-y=w176:i32)
            n64 = property class="Auto Track Wave.lvclass"(reference=refnum<class "Auto Track Wave.lvclass"> refnum ("Auto Tracking Wave.lvclass"), "Accessors:slope length"=w189, "Accessors:slope type"=w188) -> (reference out=w183:refnum<class "Auto Track Wave.lvclass">, error out=w182:errorcluster)  [unwired: 1 in]
          }
          frame 5 {
            n65 = Subtract(x=w194, y=36) -> (x-y=w192:i32)
            n66 = Subtract(x=w193, y=36) -> (x-y=w191:i32)
            n67 = property class="Auto Brake (Square) Wave.lvclas"(reference=refnum<class "Auto Brake (Square) Wave.lvclass"> refnum ("Auto Braking Wave.lvclass"), "Accessors:slope length"=w204, "Accessors:slope type"=w203) -> (reference out=w198:refnum<class "Auto Brake (Square) Wave.lvclass">, error out=w197:errorcluster)  [unwired: 1 in]
          }
          frame 6 {
            n68 = Add(x=w210, y=84) -> (x+y=w208:i32)
            n69 = Add(x=w209, y=84) -> (x+y=w207:i32)
          }
          frame 7 {
            n70 = Add(x=w220, y=84) -> (x+y=w218:i32)
            n71 = Add(x=w216, y=84) -> (x+y=w215:i32)
          }
        }
        n72 = Not(x=w114) -> (.not. x?=w113:bool)
        n73 = property on="Freq." class="DigNum (엄격한)"("Caption.Text"=w117) -> ()  [unwired: 2 in, 2 out]
        n74 = property on="Square_Slope Length" class="DigNum (엄격한)"("Visible"=w125, "Top"=w116) -> ()  [unwired: 2 in, 2 out]
        n75 = property on="Square_Slope" class="Enum (엄격한)"("Visible"=w124, "Top"=w115) -> ()  [unwired: 2 in, 2 out]
        n76 = property on="Scale" class="DigNum (엄격한)"("Visible"=w113) -> ()  [unwired: 2 in, 2 out]
        n77 = property on="Cycle" class="DigNum (엄격한)"("Visible"=w113) -> ()  [unwired: 2 in, 2 out]
        n78 = property on="Repeat Type" class="Enum (엄격한)"("Visible"=w113) -> ()  [unwired: 2 in, 2 out]
        n79 = local read "WF Seq_Voltage Range"() -> (w119:dbl)
        n80 = local read "WF List_Sampling Rate"() -> (w128:u32)
        n81 = local read "WF Seq_Wait"() -> (w118:u8)
        n82 = property on="WF Gen_Add to Seq" class="Bool"("DisabledEnum"=w110) -> ()  [unwired: 2 in, 2 out]
        n83 = property on="WF Gen_Change" class="Bool"("DisabledEnum"=w110) -> ()  [unwired: 2 in, 2 out]
        n84 = property class="Waveform Gen.lvclass"(reference=w134, error in=w133, "Accessors:frequency"=w132, "Accessors:scale"=w131, "Accessors:cycle"=w130, "Accessors:repeat type"=w129, "Accessors:sampling rate"=w128, "Accessors:voltage range"=w119, "Accessors:wait"=w118) -> (reference out=w121:refnum<class "Waveform Gen.lvclass">)  [unwired: 1 out]
      }
      event "WF Gen_Add to Seq": Value Change {
        # "WF Seq 리스트박스에 표시될 파형 이름 추가"
        # "Waveform Gen 클래스 객체 데이터를\nWF Seq 배열에 추가"
        n85 = event-data() -> ()  [unwired: 1 in, 6 out]
        n86 = Generate User Event(user event=w226, event data cluster=(Ctrl)Waveform_Editor_Update_Graph_User_Event."WF Seq" ("이벤트 데이터")) -> ()  [unwired: 2 in, 2 out]
        n87 = Generate User Event(user event=w225, event data cluster=(Ctrl)Waveform_Editor_Update_Listbox_User_Event."WF Seq" ("이벤트 데이터")) -> ()  [unwired: 2 in, 2 out]
        n88 = call-dynamic "set name.vi"("Waveform Obj 입력"=w223) -> ("Waveform Obj 출력"=w229:refnum<class "Waveform Obj.lvclass">)  [unwired: 9 in, 1 out]
        n89 = Build Array (concatenate)(w231, w229) -> (w230:refnum<class "Waveform Obj.lvclass">[])
      }
      event "WF Gen_Change": Value Change {
        n90 = event-data() -> ()  [unwired: 1 in, 6 out]
        n91 = Generate User Event(user event=w235, event data cluster=(Ctrl)Waveform_Editor_Update_Graph_User_Event."WF Seq" ("이벤트 데이터")) -> ()  [unwired: 2 in, 2 out]
        n92 = Generate User Event(user event=w234, event data cluster=(Ctrl)Waveform_Editor_Update_Listbox_User_Event."WF Seq" ("이벤트 데이터")) -> ()  [unwired: 2 in, 2 out]
        n93 = local read "WF Seq"() -> (w239:i32[])
        n94 = disable-structure shown="활성화" {
          disable-tunnel: w241 -> [w245 w259]
          disable-tunnel: [w244 w256] -> w240
          disable-tunnel: w239 -> [w243 w257]
          disable-tunnel: w238 -> [w242 w258]
          disable-tunnel: [w242 w255] -> w232
          frame Disabled {
            n95 = for {
              shift-right: [w246] -> w244
              shift-left: w245 -> [w249]
              tunnel: w243 -> [w248] mode=indexing
              tunnel: w242 -> [w247]
              n96 = in-place {
                in-place-border: w247 -> [w253]
                n97 = in-place-array #2(w249, w248) -> (w254:refnum<class "Waveform Obj.lvclass">)
                n98 = property class="Waveform Obj.lvclass"(reference=w254) -> (error out=w252:errorcluster, "Accessors:name"=w251:string)  [unwired: 1 in, 1 out]
                n99 = property class="Waveform Obj.lvclass"(reference=w253, error in=w252, "Accessors:name"=w251) -> (reference out=w250:refnum<class "Waveform Obj.lvclass">)  [unwired: 1 out]
                n100 = in-place-array #2(w250) -> (w246:refnum<class "Waveform Obj.lvclass">[])  [unwired: 1 out]
              }
            }
          }
          frame Enabled {
            # "WF Seq 리스트박스에서 선택한 객체를 대체"
            n101 = call-dynamic "set name.vi"("Waveform Obj 입력"=w258) -> ("Waveform Obj 출력"=w255:refnum<class "Waveform Obj.lvclass">)  [unwired: 9 in, 1 out]
            n102 = for {
              shift-right: [w260] -> w256
              shift-left: w259 -> [w263]
              tunnel: w255 -> [w262]
              tunnel: w257 -> [w261] mode=indexing
              n103 = Replace Array Subset(array=w263, new element=w262, index=w261) -> (w260:refnum<class "Waveform Obj.lvclass">[])
            }
          }
        }
      }
      event "WF Seq_View": Value Change {
        # "WF Seq 배열로 만들어진 파형 보기"
        n104 = event-data() -> ()  [unwired: 1 in, 6 out]
        n105 = Generate User Event(user event=w266, event data cluster=(Ctrl)Waveform_Editor_Update_Graph_User_Event."WF Seq" ("이벤트 데이터")) -> ()  [unwired: 2 in, 2 out]
      }
      event "WF Seq_Up": Value Change {
        # "WF Seq 배열 순서 변경"
        n106 = event-data() -> ()  [unwired: 1 in, 6 out]
        n107 = local read "WF Seq"() -> (w277:i32[])
        n108 = Generate User Event(user event=w271, event data cluster=(Ctrl)Waveform_Editor_Update_Graph_User_Event."WF Seq" ("이벤트 데이터")) -> ()  [unwired: 2 in, 2 out]
        n109 = Generate User Event(user event=w270, event data cluster=(Ctrl)Waveform_Editor_Update_Listbox_User_Event."WF Seq" ("이벤트 데이터")) -> ()  [unwired: 2 in, 2 out]
        n110 = for {
          tunnel: w277 -> [w281] mode=indexing
          shift-right: [w283] -> w275
          shift-left: w276 -> [w284]
          tunnel: [w279] -> w274 mode=indexing
          i -> [w282]
          n111 = Equal?(x=w281, y=w282) -> (x = y?=w280:bool)
          n112 = case shown="거짓" w280 {
            tunnel: w284 -> [w290 w292]
            tunnel: w281 -> [w288 w291]
            tunnel: [w286 w292] -> w283
            tunnel: [w285 w291] -> w279
            frame False {
              n113 = Delete From Array(array=w290, index=w288) -> (deleted portion=w287:refnum<class "Waveform Obj.lvclass">, array with subset deleted=w289:refnum<class "Waveform Obj.lvclass">[])  [unwired: 1 in]
              n114 = Decrement(x=w288) -> (x-1=w285:i32)
              n115 = Insert Into Array(array=w289, index=w285, new element=w287) -> (w286:refnum<class "Waveform Obj.lvclass">[])
            }
            frame True {
            }
          }
        }
        n116 = local write "WF Seq"(w274) -> ()
      }
      event "WF Seq_Down": Value Change {
        # "WF Seq 배열 순서 변경"
        n117 = event-data() -> ()  [unwired: 1 in, 6 out]
        n118 = local read "WF Seq"() -> (w302:i32[])
        n119 = Generate User Event(user event=w295, event data cluster=(Ctrl)Waveform_Editor_Update_Graph_User_Event."WF Seq" ("이벤트 데이터")) -> ()  [unwired: 2 in, 2 out]
        n120 = Generate User Event(user event=w294, event data cluster=(Ctrl)Waveform_Editor_Update_Listbox_User_Event."WF Seq" ("이벤트 데이터")) -> ()  [unwired: 2 in, 2 out]
        n121 = Reverse 1D Array(array=w302) -> (reversed array=w303:i32[])
        n122 = Array Size(array=w299) -> (size(s)=w301:i32)
        n123 = Decrement(x=w301) -> (x-1=w300:i32)
        n124 = for {
          tunnel: w303 -> [w312] mode=indexing
          shift-right: [w313] -> w305
          shift-left: w299 -> [w314]
          tunnel: [w310] -> w304 mode=indexing
          tunnel: w300 -> [w308]
          i -> [w309]
          n125 = Subtract(x=w308, y=w309) -> (x-y=w307:i32)
          n126 = Equal?(x=w312, y=w307) -> (x = y?=w311:bool)
          n127 = case shown="거짓" w311 {
            tunnel: w314 -> [w320 w322]
            tunnel: w312 -> [w318 w321]
            tunnel: [w316 w322] -> w313
            tunnel: [w315 w321] -> w310
            frame False {
              n128 = Delete From Array(array=w320, index=w318) -> (deleted portion=w317:refnum<class "Waveform Obj.lvclass">, array with subset deleted=w319:refnum<class "Waveform Obj.lvclass">[])  [unwired: 1 in]
              n129 = Increment(x=w318) -> (x+1=w315:i32)
              n130 = Insert Into Array(array=w319, index=w315, new element=w317) -> (w316:refnum<class "Waveform Obj.lvclass">[])
            }
            frame True {
            }
          }
        }
        n131 = call "Sort 1D Array.vim"("unsorted array"=w304) -> ("sorted array"=w298:i32[])  [unwired: 10 in]
        n132 = local write "WF Seq"(w298) -> ()
      }
      event "WF Seq_Rename": Value Change {
        # "WF Seq 배열 내 파형 이름을 바꾸기 위해\n리스트박스 편집 활성화"
        n133 = event-data() -> ()  [unwired: 1 in, 6 out]
        n134 = local read "WF Seq"() -> (w328:i32[])
        n135 = Index Array(array=w328) -> (element=w326:i32)  [unwired: 1 in]
        n136 = Bundle(w326, "Column"=0) -> (w324:cluster{i32, "Column":i32})  [unwired: 1 in]
        n137 = property on="WF Seq" class="MCListbox (엄격한)"("Key Focus"=TRUE ("키 포커스"), "EditPos"=w324) -> ()  [unwired: 2 in, 2 out]
      }
      event "WF Seq": Edit Cell {
        # "WF Seq 셀을 편집하면 해당 파형의 이름을 수정"
        n138 = event-data() -> ("String"=w335:string, "Coords"=w337:T21)  [unwired: 1 in, 4 out]
        n139 = Unbundle By Name(w337) -> ("Row"=w336:i32)
        n140 = Generate User Event(user event=w332, event data cluster=(Ctrl)Waveform_Editor_Update_Listbox_User_Event."WF Seq" ("이벤트 데이터")) -> ()  [unwired: 2 in, 2 out]
        n141 = in-place {
          in-place-border: w335 -> [w340]
          n142 = in-place-array #3(w338, w336) -> (w342:refnum<class "Waveform Obj.lvclass">)
          n143 = property class="Waveform Obj.lvclass"(reference=w342, "Accessors:name"=w340) -> (reference out=w341:refnum<class "Waveform Obj.lvclass">)  [unwired: 1 in, 1 out]
          n144 = in-place-array #3(w341) -> (w334:refnum<class "Waveform Obj.lvclass">[])  [unwired: 1 out]
        }
      }
      event "WF Seq_Delete": Value Change {
        # "WF Seq 리스트박스에서 선택한 파형들을 삭제"
        n145 = event-data() -> ()  [unwired: 1 in, 6 out]
        n146 = Generate User Event(user event=w346, event data cluster=(Ctrl)Waveform_Editor_Update_Graph_User_Event."WF Seq" ("이벤트 데이터")) -> ()  [unwired: 2 in, 2 out]
        n147 = Generate User Event(user event=w345, event data cluster=(Ctrl)Waveform_Editor_Update_Listbox_User_Event."WF Seq" ("이벤트 데이터")) -> ()  [unwired: 2 in, 2 out]
        n148 = local read "WF Seq"() -> (w344:i32[])
        n149 = Reverse 1D Array(array=w344) -> (reversed array=w350:i32[])
        n150 = for {
          tunnel: w350 -> [w354] mode=indexing
          shift-right: [w353] -> w349
          shift-left: w351 -> [w355]
          n151 = Delete From Array(array=w355, index=w354) -> (array with subset deleted=w353:refnum<class "Waveform Obj.lvclass">[])  [unwired: 1 in, 1 out]
        }
      }
      event "WF Seq_Save File": Value Change {
        # "WF Seq 배열을 XML 파일로 저장\n\n이 이벤트 케이스는 현재 사용하지 않음"
        n152 = event-data() -> ()  [unwired: 1 in, 6 out]
        n153 = call "파일 대화 상자"("prompt"="Save waveform sequence...", "pattern (all files)"="*.xml", "pattern label"="Waveform Seq.") -> ("selected path"=w360:path, "cancelled"=w363:bool, "error out"=w361:errorcluster)  [unwired: 9 in, 1 out]
        n154 = Or(x=w363, y=w361) -> (x .or. y?=w362:bool)
        n155 = case shown="거짓" w362 {
          tunnel: w358 -> [w366 _]
          tunnel: w360 -> [w373 _]
          frame False {
            n156 = Open/Create/Replace File(file path (use dialog)=w373, operation (0:open)=T16."replace or create" ("동작(0:open)")) -> (refnum out=w369:refnum<file>, error out=w368:errorcluster)  [unwired: 4 in, 1 out]
            n157 = Flatten To XML(6:w366) -> (2:w372:string)
            n158 = Write to Text File(file (use dialog)=w369, text=w372, error in=w368) -> (refnum out=w371:refnum<file>, error out=w370:errorcluster)  [unwired: 1 in, 1 out]
            n159 = Close File(refnum=w371, error in=w370) -> ()  [unwired: 2 out]
          }
          frame True {
          }
        }
      }
      event "WF Seq_Load File": Value Change {
        # "WF Seq 배열을 저장한 XML 파일 불러오기\n\n이 이벤트 케이스는 현재 사용하지 않음"
        n160 = event-data() -> ()  [unwired: 1 in, 6 out]
        n161 = Generate User Event(user event=w380, event data cluster=(Ctrl)Waveform_Editor_Update_Graph_User_Event."WF Seq" ("이벤트 데이터")) -> ()  [unwired: 2 in, 2 out]
        n162 = Generate User Event(user event=w379, event data cluster=(Ctrl)Waveform_Editor_Update_Listbox_User_Event."WF Seq" ("이벤트 데이터")) -> ()  [unwired: 2 in, 2 out]
        n163 = call "파일 대화 상자2"("prompt"="Open waveform sequence...", "pattern (all files)"="*.xml", "pattern label"="Waveform Seq.") -> ("selected path"=w383:path, "cancelled"=w386:bool, "error out"=w384:errorcluster)  [unwired: 9 in, 1 out]
        n164 = Or(x=w386, y=w384) -> (x .or. y?=w385:bool)
        n165 = case shown="거짓" w385 {
          tunnel: w383 -> [w404 _]
          tunnel: w377 -> [w390 w411]
          tunnel: [w389 w411] -> w376
          frame False {
            n166 = Open/Create/Replace File(file path (use dialog)=w404, operation (0:open)=T16."open" ("동작(0:open)")) -> (refnum out=w401:refnum<file>, error out=w400:errorcluster)  [unwired: 4 in, 1 out]
            n167 = local read "WF List_Sampling Rate"() -> (w393:u32)
            n168 = Read from Text File(file (use dialog)=w401, error in=w400) -> (refnum out=w403:refnum<file>, text=w398:string, error out=w402:errorcluster)  [unwired: 2 in, 1 out]
            n169 = Close File(refnum=w403, error in=w402) -> (error out=w397:errorcluster)  [unwired: 1 out]
            n170 = Unflatten From XML(xml string=w398, type=refnum<class "Waveform Gen.lvclass">[] [] ("배열"), error in (no error)=w397) -> (value=w394:refnum<class "Waveform Gen.lvclass">[], error out=w395:errorcluster)
            n171 = for {
              tunnel: [w408] -> w391 mode=indexing
              tunnel: w394 -> [w407] mode=indexing
              shift-right: [w409] -> w392
              shift-left: w395 -> [w410]
              tunnel: w393 -> [w406]
              n172 = property class="Waveform Gen.lvclass"(reference=w407, error in=w410, "Accessors:sampling rate"=w406) -> (reference out=w408:refnum<class "Waveform Gen.lvclass">, error out=w409:errorcluster)
            }
            n173 = Select(t=w390, s=w392, f=w391) -> (s? t:f=w389:refnum<class "Waveform Obj.lvclass">[])
            n174 = case shown="에러 .." w392 {
              frame No Error {
              }
              frame Error {
                n175 = One Button Dialog(message="File error." ("메시지")) -> ()  [unwired: 1 in, 1 out]
              }
            }
          }
          frame True {
          }
        }
      }
      event "WF Seq": Double Click {
        # "WF Seq 리스트박스에서 특정 객체를 더블 클릭 시\n해당 객체의 데이터를 WF Gen_Setting 클러스터 컨트롤에 입력\n\n그래프 업데이트를 위해 값(신호) 프로퍼티로 이벤트 발생시킴"
        n176 = event-data() -> ("Coords"=w420:T22)  [unwired: 1 in, 8 out]
        n177 = invoke on="WF Seq" class="MCListbox (엄격한)" method="Point To Row Column"("Point"=w420) -> ("CellPosition"=w419:T21)  [unwired: 6 in, 6 out]
        n178 = property on="WF Seq" class="MCListbox (엄격한)"() -> ("RowHdrs[]"=w416:string[])  [unwired: 2 in, 2 out]
        n179 = Array Size(array=w416) -> (size(s)=w415:i32)
        n180 = Unbundle By Name(w419) -> ("Row"=w414:i32)
        n181 = In Range and Coerce(upper limit=w415, x=w414, lower limit=0 ("하위 리미트")) -> (In Range?=w412:bool)  [unwired: 1 out]
        n182 = case shown="참" w412 {
          tunnel: w418 -> [w439 _]
          tunnel: w414 -> [w438 _]
          frame True {
            n183 = Index Array(array=w439, index=w438) -> (element=w436:refnum<class "Waveform Obj.lvclass">)
            n184 = call <vilib>:"Get LV Class Name.vi"("object"=w436) -> ("class name"=w437:string)  [unwired: 9 in, 1 out]
            n185 = Search/Split String(string=w437, search string/char (-)="." ("검색 문자열/문자 (-)")) -> (substring before match=w435:string)  [unwired: 1 in, 2 out]
            n186 = To More Specific Class(target class=refnum<class "Waveform Gen.lvclass"> refnum ("Waveform Gen.lvclass"), reference=w436) -> (specific class reference=w423:refnum<class "Waveform Gen.lvclass">)  [unwired: 1 in, 1 out]
            n187 = property class="Waveform Gen.lvclass"(reference=w423) -> (reference out=w426:refnum<class "Waveform Gen.lvclass">, "Accessors:frequency"=w432:dbl, "Accessors:scale"=w431:dbl, "Accessors:cycle"=w430:dbl, "Accessors:repeat type"=w429:T2)  [unwired: 1 in, 1 out]
            n188 = Scan From String(input string=w435, default 1=waveform_gen_type."Sine" ("Waveform Type")) -> (output 1=w427:T12)  [unwired: 3 in, 3 out]
            n189 = local read "WF Gen_Setting"() -> (w433:T4)
            n190 = Bundle By Name(cluster=w433, "Freq."=w432, "Scale"=w431, "Cycle"=w430, "Repeat Type"=w429, "Waveform Type"=w427) -> (w425:T4)
            n191 = case shown="\"Auto Track\"" w427 {
              tunnel: w426 -> [_ w447 w453 w460 w467]
              tunnel: w425 -> [w440 w444 w450 w457 w464]
              tunnel: [w440 w441 w448 w454 w461] -> w424
              frame "Sine", Default {
              }
              frame "Square" {
                n192 = To More Specific Class(target class=refnum<class "Square Wave.lvclass"> refnum ("Square Wave.lvclass"), reference=w447) -> (specific class reference=w445:refnum<class "Square Wave.lvclass">)  [unwired: 1 in, 1 out]
                n193 = property class="Square Wave.lvclass"(reference=w445) -> ("Accessors:slope length"=w443:u32, "Accessors:slope type"=w442:T3)  [unwired: 1 in, 2 out]
                n194 = Bundle By Name(cluster=w444, "Square_Slope Length"=w443, "Square_Slope"=w442) -> (w441:T4)
              }
              frame "PWL" {
                n195 = To More Specific Class(target class=refnum<class "PWL.lvclass"> refnum ("PWL.lvclass"), reference=w453) -> (specific class reference=w451:refnum<class "PWL.lvclass">)  [unwired: 1 in, 1 out]
                n196 = property class="PWL.lvclass" props=["Accessors:previous pwl scale", "Accessors:waveform type"](reference=w451) -> ("Accessors:previous pwl scale"=w449:dbl)  [unwired: 1 in, 3 out]
                n197 = Bundle By Name(cluster=w450, "Square_Slope Length"=w449) -> (w448:T4)
              }
              frame "Auto Track" {
                n198 = To More Specific Class(target class=refnum<class "Auto Track Wave.lvclass"> refnum ("Auto Tracking Wave.lvclass"), reference=w460) -> (specific class reference=w458:refnum<class "Auto Track Wave.lvclass">)  [unwired: 1 in, 1 out]
                n199 = property class="Auto Track Wave.lvclass"(reference=w458) -> ("Accessors:slope length"=w456:u32, "Accessors:slope type"=w455:T3)  [unwired: 1 in, 2 out]
                n200 = Bundle By Name(cluster=w457, "Square_Slope Length"=w456, "Square_Slope"=w455) -> (w454:T4)
              }
              frame "Auto Brake (Square)" {
                n201 = To More Specific Class(target class=refnum<class "Auto Brake (Square) Wave.lvclass"> refnum ("Auto Braking Wave.lvclass"), reference=w467) -> (specific class reference=w465:refnum<class "Auto Brake (Square) Wave.lvclass">)  [unwired: 1 in, 1 out]
                n202 = property class="Auto Brake (Square) Wave.lvclas"(reference=w465) -> ("Accessors:slope length"=w463:u32, "Accessors:slope type"=w462:T3)  [unwired: 1 in, 2 out]
                n203 = Bundle By Name(cluster=w464, "Square_Slope Length"=w463, "Square_Slope"=w462) -> (w461:T4)
              }
            }
            n204 = property on="WF Gen_Setting" class="Clust (엄격한)"("Val(Sgnl)"=w424) -> ()  [unwired: 2 in, 2 out]
          }
          frame False {
          }
        }
      }
      event "WF Seq_Voltage Range", "WF Seq_Wait": Value Change {
        # "이 컨트롤들은 WF Seq 밑에 있지만 WF Gen에 사용됨"
        n205 = event-data() -> ()  [unwired: 1 in, 6 out]
        n206 = Generate User Event(user event=w471, event data cluster=(Ctrl)Waveform_Editor_Update_Graph_User_Event."Latest" ("이벤트 데이터")) -> ()  [unwired: 2 in, 2 out]
        n207 = for {
          tunnel: w476 -> [w480] mode=indexing
          tunnel: [w479] -> w473 mode=indexing
          tunnel: "WF Seq_Voltage Range" -> [w478]
          tunnel: "WF Seq_Wait" -> [w477]
          n208 = property class="Waveform Obj.lvclass"(reference=w480, "Accessors:voltage range"=w478, "Accessors:wait"=w477) -> (reference out=w479:refnum<class "Waveform Obj.lvclass">)  [unwired: 1 in, 1 out]
        }
        n209 = property class="Waveform Obj.lvclass"(reference=w475, "Accessors:voltage range"="WF Seq_Voltage Range", "Accessors:wait"="WF Seq_Wait") -> (reference out=w474:refnum<class "Waveform Obj.lvclass">)  [unwired: 1 in, 1 out]
      }
      event "WF Seq_Play Mode": Value Change {
        # "현재 DW7802에만 해당하는 기능"
        n210 = event-data() -> ()  [unwired: 1 in, 6 out]
        n211 = case shown="1" "WF Seq_Play Mode" {
          tunnel: w485 -> [w497 _]
          tunnel: w483 -> [w494 _]
          tunnel: w482 -> [w490 _]
          tunnel: [w488 _] -> w481
          frame 0, Default {
            w498 = T17."Enabled" ("비활성화")
            w499 = TRUE ("보이기")
            w500 = FALSE ("보이기")
            # "일반 웨이브폼"
            n212 = Index Array(array=w490) -> (element=w493:refnum<class "Waveform Obj.lvclass">)  [unwired: 1 in]
            n213 = property class="Waveform Obj.lvclass"(reference=w493) -> ("Accessors:play mode"=w492:u8)  [unwired: 1 in, 2 out]
            n214 = Generate User Event(user event=w497, event data cluster=(Ctrl)Waveform_Editor_Update_Graph_User_Event."WF Seq" ("이벤트 데이터")) -> ()  [unwired: 2 in, 2 out]
            n215 = Generate User Event(user event=w494, event data cluster=(Ctrl)Waveform_Editor_Update_Listbox_User_Event."WF Seq" ("이벤트 데이터")) -> ()  [unwired: 2 in, 2 out]
            n216 = property on="WF Seq_PWL Listbox" class="MCListbox (엄격한)"("Visible"=w500) -> ()  [unwired: 2 in, 2 out]
            n217 = property on="WF Seq_PWL_DW7802" class="Arr (엄격한)"("Visible"=w500) -> ()  [unwired: 2 in, 2 out]
            n218 = property on="WF Seq_PWL Points" class="Ring (엄격한)"("Visible"=w500) -> ()  [unwired: 2 in, 2 out]
            n219 = Equal To 0?(x=w492) -> (x = 0?=w491:bool)
            n220 = property on="WF Seq_Up" class="Bool"("Visible"=w499) -> ()  [unwired: 2 in, 2 out]
            n221 = property on="WF Seq_Down" class="Bool"("Visible"=w499) -> ()  [unwired: 2 in, 2 out]
            n222 = property on="WF Seq_Rename" class="Bool"("Visible"=w499) -> ()  [unwired: 2 in, 2 out]
            n223 = property on="WF Seq_Delete" class="Bool"("Visible"=w499) -> ()  [unwired: 2 in, 2 out]
            n224 = Select(t=w490, s=w491, f=refnum<class "Waveform Obj.lvclass">[] []) -> (s? t:f=w488:refnum<class "Waveform Obj.lvclass">[])
            n225 = property on="WF Gen_Setting" class="Clust (엄격한)"("DisabledEnum"=w498) -> ()  [unwired: 2 in, 2 out]
            n226 = property on="WF Gen_Add to Seq" class="Bool"("DisabledEnum"=w498) -> ()  [unwired: 2 in, 2 out]
            n227 = property on="WF Gen_Change" class="Bool"("DisabledEnum"=w498) -> ()  [unwired: 2 in, 2 out]
          }
          frame 1 {
            w504 = T17."Disabled and Grayed Out" ("비활성화")
            w505 = FALSE ("보이기")
            w506 = TRUE ("보이기")
            # "PWL"
            n228 = local read "WF Seq_PWL Points"() -> (w503:u8)
            n229 = property on="WF Seq_PWL Listbox" class="MCListbox (엄격한)"("Visible"=w506) -> ()  [unwired: 2 in, 2 out]
            n230 = property on="WF Seq_PWL_DW7802" class="Arr (엄격한)"("Visible"=w506) -> ()  [unwired: 2 in, 2 out]
            n231 = property on="WF Seq_PWL Points" class="Ring (엄격한)"("Visible"=w506, "Val(Sgnl)"=w503) -> ()  [unwired: 2 in, 2 out]
            n232 = property on="WF Seq_Up" class="Bool"("Visible"=w505) -> ()  [unwired: 2 in, 2 out]
            n233 = property on="WF Seq_Down" class="Bool"("Visible"=w505) -> ()  [unwired: 2 in, 2 out]
            n234 = property on="WF Seq_Rename" class="Bool"("Visible"=w505) -> ()  [unwired: 2 in, 2 out]
            n235 = property on="WF Seq_Delete" class="Bool"("Visible"=w505) -> ()  [unwired: 2 in, 2 out]
            n236 = property on="WF Seq_View" class="Bool"("DisabledEnum"=T17."Enabled" ("비활성화")) -> ()  [unwired: 2 in, 2 out]
            n237 = property on="WF Gen_Setting" class="Clust (엄격한)"("DisabledEnum"=w504) -> ()  [unwired: 2 in, 2 out]
            n238 = property on="WF Gen_Add to Seq" class="Bool"("DisabledEnum"=w504) -> ()  [unwired: 2 in, 2 out]
            n239 = property on="WF Gen_Change" class="Bool"("DisabledEnum"=w504) -> ()  [unwired: 2 in, 2 out]
            n240 = property on="WF Seq_Add to List" class="Bool"("DisabledEnum"=T17."Enabled" ("비활성화")) -> ()  [unwired: 2 in, 2 out]
          }
        }
      }
      event "WF Seq_PWL Points": Value Change {
        # "현재 DW7802에만 해당하는 기능"
        n241 = event-data() -> ()  [unwired: 1 in, 6 out]
        n242 = local read "WF Seq_PWL_DW7802"() -> (w512:T1)
        n243 = To Long Integer(number="WF Seq_PWL Points") -> (32bit integer=w507:i32)
        n244 = Array Size(array=w512) -> (size(s)=w508:i32)
        n245 = Subtract(x=w507, y=w508) -> (x-y=w511:i32)
        n246 = for {
          N: w507 -> [_]
          tunnel: [w529] -> w514 mode=indexing
          i -> [w530]
          n247 = Increment(x=w530) -> (x+1=w529:i32)
        }
        n248 = case shown="1.." w511 {
          selector: w511 -> [_ _ w526]
          tunnel: w512 -> [w520 w521 w525]
          tunnel: [w518 w521 w523] -> w510
          tunnel: w507 -> [w519 _ _]
          tunnel: w508 -> [_ _ w528]
          frame ..-1 {
            # "PWL 포인트 수를 줄임"
            n249 = Array Subset(array=w520, length=w519) -> (w518:T1)  [unwired: 1 in]
          }
          frame 0 {
            # "PWL 포인트 수 변경 x"
          }
          frame 1.. {
            # "PWL Point 수를 늘림"
            n250 = Decrement(x=w528) -> (x-1=w522:i32)
            n251 = Index Array(array=w525, index=w522) -> (element=w527:T23)
            n252 = Initialize Array(w527, w526) -> (w524:T1)
            n253 = Build Array (concatenate)(w525, w524) -> (w523:T1)
          }
        }
        n254 = Number To Decimal String(number=w514) -> (decimal integer string=w513:string[])  [unwired: 1 in]
        n255 = property on="WF Seq_PWL_DW7802" class="Arr (엄격한)"("Number of Rows"=w507, "Val(Sgnl)"=w510) -> ()  [unwired: 2 in, 2 out]
        n256 = property on="WF Seq_PWL Listbox" class="MCListbox (엄격한)"("RowHdrs[]"=w513) -> ()  [unwired: 2 in, 2 out]
      }
      event "WF Seq_PWL_DW7802": Value Change {
        # "현재 DW7802에만 해당하는 기능"
        # "PWL 설정에 따라 Waveform Gen 클래스를 상속받는 \nPWL 클래스 객체 배열 생성"
        n257 = event-data() -> ()  [unwired: 1 in, 6 out]
        n258 = Generate User Event(user event=w534, event data cluster=(Ctrl)Waveform_Editor_Update_Graph_User_Event."WF Seq" ("이벤트 데이터")) -> ()  [unwired: 2 in, 2 out]
        n259 = for {
          tunnel: "WF Seq_PWL_DW7802" -> [w553] mode=indexing
          tunnel: [w542] -> w536 mode=indexing
          shift-right: [w544] -> _
          shift-left: 0.0 ("Amplitude") -> [w543]
          tunnel: [w541] -> w532 mode=concatenating
          n260 = Unbundle By Name(w553) -> ("Shape"=w552:u16, "Ramp"=w551:u16, "Amplitude"=w544:dbl, "Frequency"=w550:dbl, "Cycle"=w549:dbl)
          n261 = local read "WF Seq_Play Mode"() -> (w547:u8)
          n262 = local read "WF List_Sampling Rate"() -> (w546:u32)
          n263 = local read "WF Seq_Voltage Range"() -> (w545:dbl)
          n264 = property class="PWL_DW7802.lvclass"(reference=refnum<class "PWL_DW7802.lvclass"> refnum ("PWL_DW7802.lvclass"), "Accessors:waveform type"=w552, "Accessors:repeat type"=w551, "Accessors:scale"=w544, "Accessors:frequency"=w550, "Accessors:cycle"=w549, "Accessors:play mode"=w547, "Accessors:sampling rate"=w546, "Accessors:voltage range"=w545, "Accessors:previous pwl scale"=w543) -> (reference out=w548:refnum<class "PWL_DW7802.lvclass">)  [unwired: 1 in, 1 out]
          n265 = call-dynamic "get waveform - 8bit.vi"("PWL_DW7802 입력"=w548) -> ("8bit memory data"=w541:u8[], "PWL_DW7802 출력"=w542:refnum<class "PWL_DW7802.lvclass">)  [unwired: 7 in, 2 out]
        }
        n266 = Array Size(array=w532) -> (size(s)=w531:i32)
        n267 = local write "WF Seq_Total Bytes"(w531) -> ()
      }
      event "WF Seq_Add to List": Value Change {
        # "Waveform 클래스 객체 배열을 클러스터화 해서\nWF List 배열에 추가"
        n268 = event-data() -> ()  [unwired: 1 in, 6 out]
        n269 = Generate User Event(user event=w554, event data cluster=(Ctrl)Waveform_Editor_Update_Listbox_User_Event."WF List" ("이벤트 데이터")) -> ()  [unwired: 2 in, 2 out]
        n270 = local read "WF List_Sampling Rate"() -> (w556:u32)
        n271 = call "(SubVI)Waveform Editor_Build WF Seq.vi"("Sampling Rate"=w556, "WF Seq"=w558) -> ("WF List Elements"=w557:T9)  [unwired: 4 in, 5 out]
        n272 = Build Array (concatenate)(w560, w557) -> (w559:T9[])
      }
      event "WF Seq_Change": Value Change {
        # "WF List 리스트박스에서 선택한 객체를 대체"
        n273 = event-data() -> ()  [unwired: 1 in, 6 out]
        n274 = Generate User Event(user event=w568, event data cluster=(Ctrl)Waveform_Editor_Update_Listbox_User_Event."WF List" ("이벤트 데이터")) -> ()  [unwired: 2 in, 2 out]
        n275 = local read "WF List_Sampling Rate"() -> (w564:u32)
        n276 = call "(SubVI)Waveform Editor_Build WF Seq.vi"("Sampling Rate"=w564, "WF Seq"=w563) -> ("WF List Elements"=w562:T9)  [unwired: 4 in, 5 out]
        n277 = local read "WF List"() -> (w566:i32[])
        n278 = disable-structure shown="활성화" {
          disable-tunnel: w567 -> [w574 w586]
          disable-tunnel: w566 -> [w573 w584]
          disable-tunnel: [w572 w585] -> w565
          disable-tunnel: w562 -> [w571 w583]
          frame Disabled {
            n279 = for {
              tunnel: w573 -> [w577] mode=indexing
              shift-right: [w576] -> w572
              shift-left: w574 -> [w578]
              tunnel: w571 -> [w575]
              n280 = in-place {
                in-place-border: w575 -> [w579]
                n281 = in-place-array #4(w578, w577) -> (w582:T9)
                n282 = Unbundle By Name(w582) -> ("Name"=w581:string)
                n283 = Bundle By Name(cluster=w579, "Name"=w581) -> (w580:T9)
                n284 = in-place-array #4(w580) -> (w576:T9[])  [unwired: 1 out]
              }
            }
          }
          frame Enabled {
            n285 = for {
              tunnel: w584 -> [w588] mode=indexing
              shift-right: [w589] -> w585
              shift-left: w586 -> [w590]
              tunnel: w583 -> [w587]
              n286 = Replace Array Subset(array=w590, new element=w587, index=w588) -> (w589:T9[])
            }
          }
        }
      }
      event "WF List": Value Change {
        # "리스트박스에서 마지막 객체를 선택 후 Delete하면\n리스트박스의 값이 유지되는 문제가 있어서\n행 헤더 크기와 비교"
        # "48kHz까지만 RTP 지원"
        n287 = event-data() -> ()  [unwired: 1 in, 6 out]
        n288 = local read "WF List_Sampling Rate"() -> (w596:u32)
        n289 = property on="WF List" class="MCListbox (엄격한)"() -> ("RowHdrs[]"=w603:string[])  [unwired: 2 in, 2 out]
        n290 = Index Array(array="WF List") -> (element=w592:i32)  [unwired: 1 in]
        n291 = Array Size(array=w603) -> (size(s)=w601:i32)
        n292 = Array Size(array="WF List") -> (size(s)=w600:i32)
        n293 = Less?(x=w592, y=w601) -> (x < y?=w599:bool)
        n294 = Less Or Equal?(x=w596, y=u32 48000) -> (x <= y?=w593:bool)
        n295 = And(x=w599, y=w593) -> (x .and. y?=w594:bool)
        n296 = Select(t=w600, s=w594, f=0) -> (s? t:f=w597:i32)
        n297 = case shown="1" w597 {
          tunnel: [T17."Disabled and Grayed Out" ("비활성화") w610] -> w604
          tunnel: w592 -> [_ w616]
          tunnel: w591 -> [_ w617]
          frame 0, Default {
            # "리스트박스에서 선택하지 않거나\n2개 이상 선택하는 경우 RTP Start 버튼 비활성화"
          }
          frame 1 {
            # "PWL인 경우 RTP 사용 불가"
            n298 = Index Array(array=w617, index=w616) -> (element=w615:T9)
            n299 = Unbundle By Name(w615) -> ("WF Seq"=w614:refnum<class "Waveform Obj.lvclass">[])
            n300 = Index Array(array=w614) -> (element=w613:refnum<class "Waveform Obj.lvclass">)  [unwired: 1 in]
            n301 = property class="Waveform Obj.lvclass"(reference=w613) -> ("Accessors:play mode"=w612:u8)  [unwired: 1 in, 2 out]
            n302 = Equal To 0?(x=w612) -> (x = 0?=w611:bool)
            n303 = Select(t=T17."Enabled" ("비활성화"), s=w611, f=T17."Disabled and Grayed Out") -> (s? t:f=w610:T17)
          }
        }
        n304 = property on="WF List_RTP Start" class="Bool"("DisabledEnum"=w604) -> ()  [unwired: 2 in, 2 out]
      }
      event "WF List_View": Value Change {
        # "Not used"
        n305 = event-data() -> ()  [unwired: 1 in, 6 out]
        n306 = disable-structure shown="비활성화" {
          disable-tunnel: w619 -> [w623 _]
          frame Disabled {
            n307 = Generate User Event(user event=w623, event data cluster=(Ctrl)Waveform_Editor_Update_Graph_User_Event."WF List" ("이벤트 데이터")) -> ()  [unwired: 2 in, 2 out]
          }
          frame Enabled {
          }
        }
      }
      event "WF List_Up": Value Change {
        # "WF List 배열 순서 변경"
        n308 = event-data() -> ()  [unwired: 1 in, 6 out]
        n309 = local read "WF List"() -> (w630:i32[])
        n310 = Generate User Event(user event=w624, event data cluster=(Ctrl)Waveform_Editor_Update_Listbox_User_Event."WF List" ("이벤트 데이터")) -> ()  [unwired: 2 in, 2 out]
        n311 = for {
          tunnel: w630 -> [w634] mode=indexing
          shift-right: [w636] -> w627
          shift-left: w628 -> [w637]
          tunnel: [w632] -> w629 mode=indexing
          i -> [w635]
          n312 = Equal?(x=w634, y=w635) -> (x = y?=w633:bool)
          n313 = case shown="거짓" w633 {
            tunnel: w637 -> [w643 w645]
            tunnel: w634 -> [w641 w644]
            tunnel: [w639 w645] -> w636
            tunnel: [w638 w644] -> w632
            frame False {
              n314 = Delete From Array(array=w643, index=w641) -> (deleted portion=w640:T9, array with subset deleted=w642:T9[])  [unwired: 1 in]
              n315 = Decrement(x=w641) -> (x-1=w638:i32)
              n316 = Insert Into Array(array=w642, index=w638, new element=w640) -> (w639:T9[])
            }
            frame True {
            }
          }
        }
        n317 = local write "WF List"(w629) -> ()
      }
      event "WF List_Down": Value Change {
        # "WF List 배열 순서 변경"
        n318 = event-data() -> ()  [unwired: 1 in, 6 out]
        n319 = local read "WF List"() -> (w654:i32[])
        n320 = Generate User Event(user event=w646, event data cluster=(Ctrl)Waveform_Editor_Update_Listbox_User_Event."WF List" ("이벤트 데이터")) -> ()  [unwired: 2 in, 2 out]
        n321 = Reverse 1D Array(array=w654) -> (reversed array=w655:i32[])
        n322 = Array Size(array=w650) -> (size(s)=w653:i32)
        n323 = Decrement(x=w653) -> (x-1=w652:i32)
        n324 = for {
          tunnel: w655 -> [w663] mode=indexing
          shift-right: [w664] -> w649
          shift-left: w650 -> [w665]
          tunnel: [w661] -> w656 mode=indexing
          tunnel: w652 -> [w659]
          i -> [w660]
          n325 = Subtract(x=w659, y=w660) -> (x-y=w658:i32)
          n326 = Equal?(x=w663, y=w658) -> (x = y?=w662:bool)
          n327 = case shown="거짓" w662 {
            tunnel: w665 -> [w671 w673]
            tunnel: w663 -> [w669 w672]
            tunnel: [w667 w673] -> w664
            tunnel: [w666 w672] -> w661
            frame False {
              n328 = Delete From Array(array=w671, index=w669) -> (deleted portion=w668:T9, array with subset deleted=w670:T9[])  [unwired: 1 in]
              n329 = Increment(x=w669) -> (x+1=w666:i32)
              n330 = Insert Into Array(array=w670, index=w666, new element=w668) -> (w667:T9[])
            }
            frame True {
            }
          }
        }
        n331 = call "Sort 1D Array.vim"("unsorted array"=w656) -> ("sorted array"=w651:i32[])  [unwired: 10 in]
        n332 = local write "WF List"(w651) -> ()
      }
      event "WF List_Rename": Value Change {
        # "WF List 배열 내 이름을 바꾸기 위해\n리스트박스 편집 활성화"
        n333 = event-data() -> ()  [unwired: 1 in, 6 out]
        n334 = local read "WF List"() -> (w679:i32[])
        n335 = Index Array(array=w679) -> (element=w677:i32)  [unwired: 1 in]
        n336 = Bundle(w677, "Column"=0) -> (w675:cluster{i32, "Column":i32})  [unwired: 1 in]
        n337 = property on="WF List" class="MCListbox (엄격한)"("Key Focus"=TRUE ("키 포커스"), "EditPos"=w675) -> ()  [unwired: 2 in, 2 out]
      }
      event "WF List": Edit Cell {
        # "WF Seq 셀을 편집하면 해당 파형의 이름을 수정"
        n338 = event-data() -> ("String"=w687:string, "Coords"=w689:T21)  [unwired: 1 in, 4 out]
        n339 = Unbundle By Name(w689) -> ("Row"=w688:i32)
        n340 = Generate User Event(user event=w685, event data cluster=(Ctrl)Waveform_Editor_Update_Listbox_User_Event."WF List" ("이벤트 데이터")) -> ()  [unwired: 2 in, 2 out]
        n341 = in-place {
          in-place-border: w687 -> [w691]
          n342 = in-place-array #5(w683, w688) -> (w692:T9)
          n343 = Bundle By Name(cluster=w692, "Name"=w691) -> (w693:T9)
          n344 = in-place-array #5(w693) -> (w682:T9[])  [unwired: 1 out]
        }
      }
      event "WF List_Delete": Value Change {
        # "WF Seq 리스트박스에서 선택한 파형들을 삭제"
        n345 = event-data() -> ()  [unwired: 1 in, 6 out]
        n346 = Generate User Event(user event=w694, event data cluster=(Ctrl)Waveform_Editor_Update_Listbox_User_Event."WF List" ("이벤트 데이터")) -> ()  [unwired: 2 in, 2 out]
        n347 = local read "WF List"() -> (w699:i32[])
        n348 = Reverse 1D Array(array=w699) -> (reversed array=w700:i32[])
        n349 = for {
          tunnel: w700 -> [w703] mode=indexing
          shift-right: [w702] -> w697
          shift-left: w698 -> [w704]
          n350 = Delete From Array(array=w704, index=w703) -> (array with subset deleted=w702:T9[])  [unwired: 1 in, 1 out]
        }
      }
      event "WF List_Import": Value Change {
        n351 = event-data() -> ()  [unwired: 1 in, 6 out]
        n352 = Generate User Event(user event=w711, event data cluster=(Ctrl)Waveform_Editor_Update_Listbox_User_Event."WF List" ("이벤트 데이터")) -> ()  [unwired: 2 in, 2 out]
        n353 = disable-structure shown="활성화" {
          disable-tunnel: ["Import..." ("prompt") "Import..." ("prompt")] -> w717
          disable-tunnel: ["*.wav;*.txt" ("pattern (all files)") "*.wav" ("pattern (all files)")] -> w716
          disable-tunnel: ["wav,txt" ("pattern label") "wav" ("pattern label")] -> w706
          frame Enabled {
            # "#개발버전"
          }
          frame Disabled {
            # "#배포버전"
          }
        }
        n354 = call "파일 대화 상자6"("prompt"=w717, "pattern (all files)"=w716, "pattern label"=w706) -> ("selected path"=w708:path, "cancelled"=w715:bool, "error out"=w714:errorcluster)  [unwired: 9 in, 1 out]
        n355 = local read "WF List_Sampling Rate"() -> (w705:u32)
        n356 = Or(x=w715, y=w714) -> (x .or. y?=w713:bool)
        n357 = call <vilib>:"Get File Extension.vi"("file"=w708) -> ("lowercase file extension"=w707:string)  [unwired: 6 in, 4 out]
        n358 = case shown="거짓" w713 {
          tunnel: w708 -> [w728 _]
          tunnel: w710 -> [w730 w762]
          tunnel: [w729 w762] -> w709
          tunnel: w707 -> [w727 _]
          tunnel: w705 -> [w726 _]
          frame False {
            n359 = case shown="\"txt\", 기본" w727 {
              tunnel: w730 -> [w733 w752]
              tunnel: [w732 w751] -> w729
              tunnel: w728 -> [w736 w746]
              tunnel: w726 -> [w731 _]
              frame "txt", Default {
                n360 = call "(SubVI)Waveform Editor_Import Manager_TextFile.vi"("WF List_Sampling Rate"=w731, "File Path"=w736) -> ("Apply?"=w734:bool, "Text File 출력"=w735:refnum<class "Text File.lvclass">)  [unwired: 7 in, 1 out]
                n361 = case shown="참" w734 {
                  tunnel: [w737 w745] -> w732
                  tunnel: w735 -> [_ w743]
                  tunnel: w733 -> [w737 w738]
                  frame False {
                  }
                  frame True {
                    n362 = property class="Text File.lvclass"(reference=w743) -> (reference out=w741:refnum<class "Text File.lvclass">, "Accessors:name"=w742:string)  [unwired: 1 in, 1 out]
                    n363 = Build Array(w741) -> (w740:refnum<class "Text File.lvclass">[])
                    n364 = Bundle By Name(cluster=T9 {"Name"="", "WF Seq"=[]}, "WF Seq"=w740, "Name"=w742) -> (w739:T9)
                    n365 = Build Array (concatenate)(w738, w739) -> (w745:T9[])
                  }
                }
              }
              frame "wav" {
                n366 = local read "WF List_Sampling Rate"() -> (w748:u32)
                n367 = call "(SubVI)Waveform Editor_Import Manager.vi"("New?"=TRUE, "Sampling Rate In"=w748, "File Path"=w746) -> ("Apply?"=w749:bool, "*.WAV Data"=w750:refnum<class "WAV File.lvclass">)  [unwired: 6 in, 1 out]
                n368 = case shown="참" w749 {
                  tunnel: w752 -> [w753 w761]
                  tunnel: [w753 w760] -> w751
                  tunnel: w750 -> [_ w758]
                  frame False {
                  }
                  frame True {
                    n369 = property class="WAV File.lvclass"(reference=w758) -> (reference out=w756:refnum<class "WAV File.lvclass">, "Accessors:name"=w757:string)  [unwired: 1 in, 1 out]
                    n370 = Build Array(w756) -> (w755:refnum<class "WAV File.lvclass">[])
                    n371 = Bundle By Name(cluster=T9 {"Name"="", "WF Seq"=[]}, "WF Seq"=w755, "Name"=w757) -> (w754:T9)
                    n372 = Build Array (concatenate)(w761, w754) -> (w760:T9[])
                  }
                }
              }
            }
          }
          frame True {
          }
        }
      }
      event "WF List_Export": Value Change {
        # "파형 데이터를 txt, wav 파일로 Export"
        n373 = event-data() -> ()  [unwired: 1 in, 6 out]
        n374 = local read "WF List_Sampling Rate"() -> (w767:u32)
        n375 = property on="WF List_Mem Update" class="Bool"() -> ("Visible"=w764:bool, "DisabledEnum"=w766:T17)  [unwired: 2 in, 2 out]
        n376 = Equal To 0?(x=w766) -> (x = 0?=w765:bool)
        n377 = And(x=w764, y=w765) -> (x .and. y?=w763:bool)
        n378 = call "(SubVI)Waveform Editor_Export Manager.vi"("Enable Memory"=w763, "Sampling Rate"=w767, "WF List"=w768) -> ()  [unwired: 8 in, 1 out]
      }
      event "WF List_Save File": Value Change {
        # "WF List 배열을 xml 파일로 저장\n클래스를 수정하는 경우 LabVIEW가 버전과 수정 이력을 저장하기 때문에\nxml로 저장하면 수정 이전 버전의 클래스 데이터도 불러올 수 있음"
        n379 = event-data() -> ()  [unwired: 1 in, 6 out]
        n380 = call "파일 대화 상자3"("prompt"="Save waveform list...", "pattern (all files)"="*.xml", "pattern label"="Waveform List") -> ("selected path"=w774:path, "cancelled"=w778:bool, "error out"=w776:errorcluster)  [unwired: 9 in, 1 out]
        n381 = Or(x=w778, y=w776) -> (x .or. y?=w777:bool)
        n382 = case shown="참" w777 {
          tunnel: w773 -> [w781 _]
          tunnel: w774 -> [w788 _]
          frame False {
            n383 = Open/Create/Replace File(file path (use dialog)=w788, operation (0:open)=T16."replace or create" ("동작(0:open)")) -> (refnum out=w784:refnum<file>, error out=w783:errorcluster)  [unwired: 4 in, 1 out]
            n384 = Flatten To XML(6:w781) -> (2:w787:string)
            n385 = Write to Text File(file (use dialog)=w784, text=w787, error in=w783) -> (refnum out=w786:refnum<file>, error out=w785:errorcluster)  [unwired: 1 in, 1 out]
            n386 = Close File(refnum=w786, error in=w785) -> ()  [unwired: 2 out]
          }
          frame True {
          }
        }
      }
      event "WF List_Load File": Value Change {
        # "xml 파일로부터 WF List 배열 데이터 불러오기"
        n387 = event-data() -> ()  [unwired: 1 in, 6 out]
        n388 = Generate User Event(user event=w796, event data cluster=(Ctrl)Waveform_Editor_Update_Graph_User_Event."Latest" ("이벤트 데이터")) -> ()  [unwired: 2 in, 2 out]
        n389 = Generate User Event(user event=w795, event data cluster=(Ctrl)Waveform_Editor_Update_Listbox_User_Event."WF List" ("이벤트 데이터")) -> ()  [unwired: 2 in, 2 out]
        n390 = call "파일 대화 상자4"("prompt"="Open waveform list...", "pattern (all files)"="*.xml", "pattern label"="Waveform List") -> ("selected path"=w793:path, "cancelled"=w801:bool, "error out"=w799:errorcluster)  [unwired: 9 in, 1 out]
        n391 = Or(x=w801, y=w799) -> (x .or. y?=w800:bool)
        n392 = case shown="거짓" w800 {
          tunnel: w793 -> [w819 _]
          tunnel: w791 -> [w807 w828]
          tunnel: [w804 w828] -> w792
          frame False {
            n393 = Open/Create/Replace File(file path (use dialog)=w819, operation (0:open)=T16."open" ("동작(0:open)")) -> (refnum out=w816:refnum<file>, error out=w815:errorcluster)  [unwired: 4 in, 1 out]
            n394 = Read from Text File(file (use dialog)=w816, error in=w815) -> (refnum out=w818:refnum<file>, text=w813:string, error out=w817:errorcluster)  [unwired: 2 in, 1 out]
            n395 = Close File(refnum=w818, error in=w817) -> (error out=w812:errorcluster)  [unwired: 1 out]
            n396 = local read "WF List_Sampling Rate"() -> (w808:u32)
            n397 = Unflatten From XML(xml string=w813, type=T9[] [] ("WF List"), error in (no error)=w812) -> (value=w810:T9[], error out=w809:errorcluster)
            n398 = for {
              tunnel: w810 -> [w827] mode=indexing
              shift-right: [w821] -> w805
              shift-left: w809 -> [w823]
              tunnel: [w824] -> w806 mode=indexing
              tunnel: w808 -> [w822]
              n399 = Unbundle By Name(w827) -> ("WF Seq"=w825:refnum<class "Waveform Obj.lvclass">[], "Name"=w826:string)
              n400 = call "(SubVI)Waveform Editor_Build WF Seq.vi"("error in (no error)"=w823, "Name (empty)"=w826, "Sampling Rate"=w822, "WF Seq"=w825) -> ("error out"=w821:errorcluster, "WF List Elements"=w824:T9)  [unwired: 2 in, 4 out]
            }
            n401 = Select(t=w807, s=w805, f=w806) -> (s? t:f=w804:T9[])
            n402 = case shown="에러 없음" w805 {
              frame No Error {
              }
              frame Error {
                n403 = One Button Dialog(message="File error." ("메시지")) -> ()  [unwired: 1 in, 1 out]
              }
            }
          }
          frame True {
          }
        }
      }
      event "WF List": Double Click {
        # "WF Seq 리스트박스에서 특정 객체를 더블 클릭 시 해당 객체의 데이터가 \n\n1. Waveform Gen 클래스를 상속받는 하위 클래스면 WF Seq 리스트 박스 또는\n    PWL 관련 컨트롤이 업데이트 되도록 함\n2. Waveform File를 상속받는 하위 클래스면 Import Manager 실행"
        n404 = event-data() -> ("Coords"=w829:T22)  [unwired: 1 in, 8 out]
        n405 = invoke on="WF List" class="MCListbox (엄격한)" method="Point To Row Column"("Point"=w829) -> ("CellPosition"=w841:T21)  [unwired: 6 in, 6 out]
        n406 = property on="WF List" class="MCListbox (엄격한)"() -> ("RowHdrs[]"=w840:string[])  [unwired: 2 in, 2 out]
        n407 = Unbundle By Name(w841) -> ("Row"=w838:i32)
        n408 = Array Size(array=w840) -> (size(s)=w839:i32)
        n409 = In Range and Coerce(upper limit=w839, x=w838, lower limit=0 ("하위 리미트")) -> (In Range?=w836:bool)  [unwired: 1 out]
        n410 = case shown="참" w836 {
          tunnel: w831 -> [w853 _]
          tunnel: w838 -> [w843 _]
          tunnel: w835 -> [w849 w934]
          tunnel: [w848 w934] -> w834
          tunnel: w833 -> [w847 _]
          tunnel: w832 -> [w846 _]
          tunnel: w831 -> [w845 w933]
          tunnel: [w844 w933] -> w830
          frame True {
            # "데이터 존재"
            n411 = Index Array(array=w853, index=w843) -> (element=w852:T9)
            n412 = Unbundle By Name(w852) -> ("WF Seq"=w850:refnum<class "Waveform Obj.lvclass">[])
            n413 = Empty Array?(array=w850) -> (empty?=w851:bool)
            n414 = case shown="거짓" w851 {
              tunnel: w850 -> [w858 _]
              tunnel: w849 -> [w861 w932]
              tunnel: [w857 w932] -> w848
              tunnel: w847 -> [w863 _]
              tunnel: w846 -> [w862 _]
              tunnel: w845 -> [w860 w930]
              tunnel: [w859 w930] -> w844
              tunnel: w843 -> [w854 _]
              frame False {
                n415 = Index Array(array=w858) -> (element=w855:refnum<class "Waveform Obj.lvclass">)  [unwired: 1 in]
                n416 = call <vilib>:"Get LV Class Name.vi"("object"=w855) -> ("class name"=w856:string)  [unwired: 9 in, 1 out]
                n417 = case shown="\"Text File.lvclass\"" w856 {
                  tunnel: w863 -> [w868 _ _ _]
                  tunnel: w862 -> [w867 _ _ _]
                  tunnel: w861 -> [_ _ w900 w920]
                  tunnel: w860 -> [w866 w877 w894 w917]
                  tunnel: [w866 w877 w891 w914] -> w859
                  tunnel: w858 -> [w865 w876 _ _]
                  tunnel: [w865 refnum<class "Waveform Obj.lvclass">[] [] ("WF Seq") w900 w920] -> w857
                  tunnel: w855 -> [_ _ w898 w919]
                  tunnel: w854 -> [_ _ w893 w916]
                  frame Default {
                    n418 = disable-structure shown="활성화" {
                      disable-tunnel: w868 -> [w872 _]
                      disable-tunnel: w867 -> [w871 _]
                      frame Disabled {
                        n419 = Generate User Event(user event=w872, event data cluster=(Ctrl)Waveform_Editor_Update_Graph_User_Event."WF Seq" ("이벤트 데이터")) -> ()  [unwired: 2 in, 2 out]
                        n420 = Generate User Event(user event=w871, event data cluster=(Ctrl)Waveform_Editor_Update_Listbox_User_Event."WF Seq" ("이벤트 데이터")) -> ()  [unwired: 2 in, 2 out]
                      }
                      frame Enabled {
                      }
                    }
                    n421 = property on="WF Seq_Play Mode" class="Ring (엄격한)"("Val(Sgnl)"=u8 0 ("값(신호)")) -> ()  [unwired: 2 in, 2 out]
                  }
                  frame "PWL.lvclass", "PWL_DW7802.lvclass" {
                    n422 = for {
                      tunnel: w876 -> [w889] mode=indexing
                      tunnel: [w882] -> w875 mode=indexing
                      tunnel: [w881] -> w873
                      tunnel: [w880] -> _
                      n423 = To More Specific Class(target class=refnum<class "PWL.lvclass"> refnum ("타겟 클래스"), reference=w889) -> (specific class reference=w880:refnum<class "PWL.lvclass">, error out=w888:errorcluster)  [unwired: 1 in]
                      n424 = property class="PWL.lvclass"(reference=w880, error in=w888) -> ("Accessors:waveform type"=w887:T12, "Accessors:repeat type"=w886:T2, "Accessors:scale"=w885:dbl, "Accessors:frequency"=w884:dbl, "Accessors:cycle"=w883:dbl, "Accessors:voltage range"=w881:dbl)  [unwired: 2 out]
                      n425 = Bundle("Accessors:waveform type"=w887, "Accessors:repeat type"=w886, "Accessors:scale"=w885, "Accessors:frequency"=w884, "Accessors:cycle"=w883) -> (w882:T24)  [unwired: 1 in]
                    }
                    n426 = property on="WF Seq_Play Mode" class="Ring (엄격한)"("Val(Sgnl)"=u8 1 ("값(신호)")) -> ()  [unwired: 2 in, 2 out]
                    n427 = Array Size(array=w875) -> (size(s)=w874:i32)
                    n428 = local write "WF Seq_PWL Points"(w874) -> ()
                    n429 = local write "WF Seq_PWL_DW7802"(w875) -> ()
                    n430 = local write "WF Seq_Voltage Range"(w873) -> ()
                  }
                  frame "WAV File.lvclass" {
                    n431 = local read "WF List_Sampling Rate"() -> (w899:u32)
                    n432 = To More Specific Class(target class=refnum<class "WAV File.lvclass"> refnum ("타겟 클래스"), reference=w898) -> (specific class reference=w897:refnum<class "WAV File.lvclass">)  [unwired: 1 in, 1 out]
                    n433 = call "(SubVI)Waveform Editor_Import Manager.vi"("Sampling Rate In"=w899, "WAV File.lvclass"=w897) -> ("Apply?"=w895:bool, "*.WAV Data"=w892:refnum<class "WAV File.lvclass">)  [unwired: 7 in, 1 out]
                    n434 = case shown="참" w895 {
                      tunnel: w894 -> [w901 w905]
                      tunnel: w893 -> [_ w904]
                      tunnel: w892 -> [_ w903]
                      tunnel: [w901 w902] -> w891
                      frame False {
                      }
                      frame True {
                        n435 = in-place {
                          in-place-border: w903 -> [w908]
                          n436 = in-place-array #6(w905, w904) -> (w909:T9)
                          n437 = Build Array(w908) -> (w907:refnum<class "WAV File.lvclass">[])
                          n438 = Bundle By Name(cluster=w909, "WF Seq"=w907) -> (w906:T9)
                          n439 = in-place-array #6(w906) -> (w902:T9[])  [unwired: 1 out]
                        }
                      }
                    }
                  }
                  frame "Text File.lvclass" {
                    n440 = local read "WF List_Sampling Rate"() -> (w912:u32)
                    n441 = To More Specific Class(target class=refnum<class "Text File.lvclass"> refnum ("Text File.lvclass"), reference=w919) -> (specific class reference=w911:refnum<class "Text File.lvclass">)  [unwired: 1 in, 1 out]
                    n442 = call "(SubVI)Waveform Editor_Import Manager_TextFile.vi"("WF List_Sampling Rate"=w912, "New?"=FALSE, "Text File.lvclass"=w911) -> ("Apply?"=w918:bool, "Text File 출력"=w915:refnum<class "Text File.lvclass">)  [unwired: 6 in, 1 out]
                    n443 = case shown="참" w918 {
                      tunnel: w917 -> [w921 w925]
                      tunnel: w916 -> [_ w924]
                      tunnel: w915 -> [_ w923]
                      tunnel: [w921 w922] -> w914
                      frame False {
                      }
                      frame True {
                        n444 = in-place {
                          in-place-border: w923 -> [w928]
                          n445 = in-place-array #7(w925, w924) -> (w929:T9)
                          n446 = Build Array(w928) -> (w927:refnum<class "Text File.lvclass">[])
                          n447 = Bundle By Name(cluster=w929, "WF Seq"=w927) -> (w926:T9)
                          n448 = in-place-array #7(w926) -> (w922:T9[])  [unwired: 1 out]
                        }
                      }
                    }
                  }
                }
              }
              frame True {
                n449 = One Button Dialog(message="No waveform sequence data." ("메시지")) -> ()  [unwired: 1 in, 1 out]
              }
            }
          }
          frame False {
          }
        }
      }
      event "WF List_Sampling Rate": Value Change {
        # "1000\n->4800\n->3000"
        # "Sampling Rate 변경에 따라 파형의 Byte 크기도 변경되므로\nWF Seq 리스트박스, WF List 리스트박스 둘 다 업데이트"
        # "WF Gen, WF Seq의 경우 그래프에 보여지는 파형 데이터만 변경하면 되므로\n클래스 속성 값만 변경\n그래프 업데이트하면 자동으로 파형 데이터가 업데이트 됨"
        # "WF List의 경우 저장, Export 등을 할 수 있기 때문에\nSampling Rate를 변경하면 다른 설정을 유지한 채 파형 데이터만 새로 생성"
        # "List Update (WF List)에서 WF_LIst 값(신호) 프로퍼티로 활성화/비활성화 되지만\nWF Build 중 버튼 클릭할 수 있어서 비활성화만 미리 함"
        n450 = event-data() -> ()  [unwired: 1 in, 6 out]
        n451 = Generate User Event(user event=w945, event data cluster=(Ctrl)Waveform_Editor_Update_Graph_User_Event."Latest" ("이벤트 데이터")) -> ()  [unwired: 2 in, 2 out]
        n452 = Generate User Event(user event=w944, event data cluster=(Ctrl)Waveform_Editor_Update_Listbox_User_Event."WF Seq" ("이벤트 데이터")) -> (user event out=w940:refnum<user-event>, error out=w941:errorcluster)  [unwired: 2 in]
        n453 = Generate User Event(user event=w940, event data cluster=(Ctrl)Waveform_Editor_Update_Listbox_User_Event."WF List" ("이벤트 데이터"), error in=w941) -> ()  [unwired: 1 in, 2 out]
        n454 = Greater?(x="WF List_Sampling Rate", y=u32 48000) -> (0:w936:bool)
        n455 = case shown="참" w936 {
          frame False {
          }
          frame True {
            n456 = property on="WF List_RTP Start" class="Bool"("DisabledEnum"=T17."Disabled and Grayed Out" ("비활성화")) -> ()  [unwired: 2 in, 2 out]
          }
        }
        n457 = for {
          tunnel: w950 -> [w959] mode=indexing
          tunnel: [w958] -> w947 mode=indexing
          tunnel: "WF List_Sampling Rate" -> [w957]
          n458 = property class="Waveform Obj.lvclass"(reference=w959, "Accessors:sampling rate"=w957) -> (reference out=w958:refnum<class "Waveform Obj.lvclass">)  [unwired: 1 in, 1 out]
        }
        n459 = for {
          tunnel: w939 -> [w953] mode=indexing
          tunnel: "WF List_Sampling Rate" -> [w954]
          tunnel: [w952] -> w938 mode=indexing
          n460 = Unbundle By Name(w953) -> ("WF Seq"=w956:refnum<class "Waveform Obj.lvclass">[], "Name"=w955:string)
          n461 = call "(SubVI)Waveform Editor_Build WF Seq.vi"("Name (empty)"=w955, "Sampling Rate"=w954, "WF Seq"=w956) -> ("WF List Elements"=w952:T9)  [unwired: 3 in, 5 out]
        }
        n462 = property class="Waveform Obj.lvclass"(reference=w949, "Accessors:sampling rate"="WF List_Sampling Rate") -> (reference out=w948:refnum<class "Waveform Obj.lvclass">)  [unwired: 1 in, 1 out]
      }
      event "WF List_Mem Update": Value Change {
        # "WF List의 파형 데이터로 메모리를 업데이트"
        n463 = event-data() -> ()  [unwired: 1 in, 6 out]
        n464 = global read "(Var)System Variables.vi" "Haptic IC"() -> (w969:refnum<class "Haptic IC.lvclass">)
        n465 = call-dynamic "set memory.vi"("WF List"=w968, "Haptic IC 입력"=w969) -> ("error out"=w967:errorcluster, "Haptic IC 출력"=w965:refnum<class "Haptic IC.lvclass">)  [unwired: 8 in]
        n466 = local read "WF List_Sampling Rate"() -> (w961:u32)
        n467 = call-dynamic "update mode in ui.vi"("error in (no error)"=w967, "mode"=(Ctrl)Mode."Memory", "Haptic IC 입력"=w965) -> ("error out"=w963:errorcluster, "Haptic IC 출력"=w960:refnum<class "Haptic IC.lvclass">)  [unwired: 7 in]
        n468 = call-dynamic "update freq in ui.vi"("error in (no error)"=w963, "sampling rate"=w961, "Haptic IC 입력"=w960) -> ("error out"=w962:errorcluster)  [unwired: 7 in, 1 out]
        n469 = case shown="에러 없음" w962 {
          tunnel: ["Update Complete" ("메시지") "Update Failed!!" ("메시지")] -> w966
          frame No Error {
          }
          frame Error {
          }
        }
        n470 = One Button Dialog(message=w966) -> ()  [unwired: 1 in, 1 out]
      }
      event "WF List_RTP Start": Value Change {
        # "rtp play core.vi에서도 stop 하기 위해\n사용자 이벤트 사용함"
        # "RTP 관련 Register 설정 후 rtp play core.vi를 비동기화 호출로 실행\nrtp play core.vi에서 RTP 데이터를 RedNoah3로 보내면서 RTP가 실행됨\n\nRTP Play 완료 시 Stop 사용자 이벤트를 발생시키기 위해 이벤트 참조 입력"
        # "#20220908\nhspark\nRTP Start 시에는 Voltage Range 변경하지 않고\n현재 Register 설정 그대로 RTP Start 하도록 요청"
        n471 = event-data() -> ()  [unwired: 1 in, 6 out]
        n472 = local read "WF List"() -> (w992:i32[])
        n473 = Index Array(array=w992) -> (element=w991:i32)  [unwired: 1 in]
        n474 = Index Array(array=w990, index=w991) -> (element=w989:T9)
        n475 = Unbundle By Name(w989) -> ("WF Seq"=w988:refnum<class "Waveform Obj.lvclass">[])
        n476 = for {
          tunnel: w988 -> [w1004] mode=indexing
          tunnel: [w1005] -> w985 mode=concatenating
          tunnel: [w1003] -> w980
          n477 = call "Read voltage range.vi"("Waveform Obj 입력"=w1004) -> ("voltage range"=w1003:dbl, "Waveform Obj 출력"=w1002:refnum<class "Waveform Obj.lvclass">)  [unwired: 8 in, 1 out]
          n478 = call-dynamic "get waveform - 8bit.vi"("Waveform Obj 입력"=w1002) -> ("8bit waveform"=w1006:waveform(i8))  [unwired: 7 in, 3 out]
          n479 = Unbundle By Name(w1006) -> ("Y"=w1005:i8[])
        }
        n480 = local read "WF List_Sampling Rate"() -> (w976:u32)
        n481 = global read "(Var)System Variables.vi" "Haptic IC"() -> (w986:refnum<class "Haptic IC.lvclass">)
        n482 = call-dynamic "rtp play.vi"("voltage range"=w980, "freq"=w976, "rtp stop event ref"=w974, "waveform data"=w985, "Haptic IC 입력"=w986) -> ("error out"=w984:errorcluster, "Haptic IC 출력"=w983:refnum<class "Haptic IC.lvclass">)  [unwired: 5 in]
        n483 = disable-structure shown="비활성화" {
          disable-tunnel: w984 -> [w999 w1000]
          disable-tunnel: w983 -> [w998 w1001]
          disable-tunnel: [w997 w1000] -> w982
          disable-tunnel: [w996 w1001] -> w981
          disable-tunnel: w980 -> [w995 _]
          frame Disabled {
            n484 = call-dynamic "update voltage range in ui.vi"("error in (no error)"=w999, "voltage range"=w995, "Haptic IC 입력"=w998) -> ("error out"=w997:errorcluster, "Haptic IC 출력"=w996:refnum<class "Haptic IC.lvclass">)  [unwired: 7 in]
          }
          frame Enabled {
          }
        }
        n485 = call-dynamic "update mode in ui.vi"("error in (no error)"=w982, "mode"=(Ctrl)Mode."RTP", "Haptic IC 입력"=w981) -> ("error out"=w977:errorcluster, "Haptic IC 출력"=w978:refnum<class "Haptic IC.lvclass">)  [unwired: 7 in]
        n486 = call-dynamic "update freq in ui.vi"("error in (no error)"=w977, "sampling rate"=w976, "Haptic IC 입력"=w978) -> ("error out"=w975:errorcluster)  [unwired: 7 in, 1 out]
        n487 = Generate User Event(user event=w974, event data cluster=TRUE ("이벤트 데이터"), error in=w975) -> ()  [unwired: 1 in, 2 out]
      }
      event "WF List_RTP Stop": Value Change {
        # "rtp play core.vi에서 RTP Stop 명령어를 보내고 \nFor 루프를 종료하도록 함"
        n488 = event-data() -> ()  [unwired: 1 in, 6 out]
        n489 = Enqueue Element(queue=w1009, element=FALSE ("원소"), error in (no error)=w1008) -> ()  [unwired: 1 in, 3 out]
      }
      event User Event {
        # "RTP Start 시 Vibration Scope에서  Scope Start 방지"
        n490 = event-data() -> ("RTP Start/Stop"=w1013:bool)  [unwired: 1 in, 4 out]
        n491 = Not(x=w1013) -> (.not. x?=w1018:bool)
        n492 = Select(t=(Ctrl)Mode_Event_Event_Type."RTP Play" ("Event Type"), s=w1013, f=(Ctrl)Mode_Event_Event_Type."RTP Stop") -> (s? t:f=w1015:T20)
        n493 = case shown="거짓" w1013 {
          tunnel: w1014 -> [w1023 _]
          frame False {
            n494 = Generate User Event(user event=w1023, event data cluster=(Ctrl)Waveform_Editor_Update_Listbox_User_Event."WF List" ("이벤트 데이터")) -> ()  [unwired: 2 in, 2 out]
          }
          frame True {
            n495 = property on="WF List_Mem Update" class="Bool"("DisabledEnum"=T17."Disabled and Grayed Out" ("비활성화")) -> ()  [unwired: 2 in, 2 out]
          }
        }
        n496 = property on="WF List_RTP Start" class="Bool"("Visible"=w1018) -> ()  [unwired: 2 in, 2 out]
        n497 = property on="WF List_RTP Stop" class="Bool"("Visible"=w1013) -> ()  [unwired: 2 in, 2 out]
        n498 = call "(SubVI)Mode Event.vi"("Event Type"=w1015) -> ()  [unwired: 9 in, 2 out]
      }
      event User Event {
        # "Latest인 경우 최근 업데이트와 동일하게"
        n499 = event-data() -> ("Update Graph"=w1029:T7)  [unwired: 1 in, 4 out]
        n500 = Not Equal?(x=w1029, y=(Ctrl)Waveform_Editor_Update_Graph_User_Event."Latest") -> (x != y?=w1028:bool)
        n501 = feedback-in #8(w1029, w1028) -> ()
        n502 = feedback #8() -> (w1027:T7)
        n503 = Select(t=w1029, s=w1028, f=w1027) -> (s? t:f=w1026:T7)
        n504 = case shown="\"WF Seq\"" w1026 {
          tunnel: w1036 -> [w1042 w1047]
          tunnel: w1035 -> [_ w1048]
          tunnel: [w1040 w1049] -> w1034
          tunnel: w1031 -> [_ _]
          tunnel: [w1038 w1047] -> w1025
          frame "WF Gen", Default {
            # "WF Gen_Setting 클러스터로 설정한 Waveform Gen 클래스 객체 데이터로 그래프 업데이트"
            n505 = call-dynamic "get waveform - voltage range scaled.vi"("Waveform Obj 입력"=w1042) -> ("scaled waveform"=w1041:waveform(dbl), "Waveform Obj 출력"=w1038:refnum<class "Waveform Obj.lvclass">)  [unwired: 8 in, 1 out]
            n506 = call <vilib>:"Get LV Class Name.vi"("object"=w1038) -> ("class name"=w1039:string)  [unwired: 9 in, 1 out]
            n507 = Unbundle By Name(w1041) -> ("Y"=w1040:dbl[])
            n508 = case shown="\"Auto Brake (Sine) Wave.lvclass\", \"Auto Brake (Square) Wave.lvclass\", \"Auto Track Wave.lvclass\"" w1039 {
              tunnel: w1038 -> [_ w1046]
              tunnel: [_ w1043] -> w1037
              frame Default {
              }
              frame "Auto Brake (Sine) Wave.lvclass", "Auto Brake (Square) Wave.lvclass", "Auto Track Wave.lvclass" {
                n509 = To More Specific Class(target class=refnum<class "Auto Track Wave.lvclass"> refnum ("Auto Tracking Wave.lvclass"), reference=w1046) -> (specific class reference=w1044:refnum<class "Auto Track Wave.lvclass">)  [unwired: 1 in, 1 out]
                n510 = call-dynamic "get tracking data info.vi"("Auto Tracking Wave 입력"=w1044) -> ("warning"=w1043:bool)  [unwired: 6 in, 4 out]
              }
            }
            n511 = property on="WF Gen_Auto Tracking Waring" class="Str"("Visible"=w1037) -> ()  [unwired: 2 in, 2 out]
          }
          frame "WF Seq" {
            # "WF Seq 배열의 Waveform Gen 클래스 객체 데이터로 만든 웨이브폼 데이터를 연결하여 그래프 업데이트"
            n512 = for {
              tunnel: w1048 -> [w1052] mode=indexing
              tunnel: [w1050] -> w1049 mode=concatenating
              n513 = call-dynamic "get waveform - voltage range scaled.vi"("Waveform Obj 입력"=w1052) -> ("scaled waveform"=w1051:waveform(dbl))  [unwired: 8 in, 2 out]
              n514 = Unbundle By Name(w1051) -> ("Y"=w1050:dbl[])
            }
          }
        }
        n515 = property on="Graph" class="WFGraph (엄격한)"("Value"=w1034) -> ("Cursor.Cursor X"=w1033:dbl, "Cursor.Cursor Y"=w1032:dbl)  [unwired: 2 in, 2 out]
        n516 = local write "Graph_Cursor X"(w1033) -> ()
        n517 = local write "Graph_Cursor Y"(w1032) -> ()
      }
      event User Event {
        n518 = event-data() -> ("Update Listbox"=w1055:T8)  [unwired: 1 in, 4 out]
        n519 = case shown="\"WF Seq\", 기본" w1055 {
          tunnel: w1054 -> [w1069 _]
          tunnel: w1053 -> [_ w1088]
          frame "WF Seq", Default {
            # "첫 실행 시 빈 배열이므로\n0 입력되는 것 방지"
            n520 = local read "WF Seq_Voltage Range"() -> (w1059:dbl)
            n521 = local read "WF Seq_Wait"() -> (w1058:u8)
            n522 = for {
              tunnel: w1069 -> [w1081] mode=indexing
              tunnel: [w1077] -> w1068 mode=indexing
              tunnel: [w1078] -> w1063 mode=indexing
              tunnel: [w1070] -> w1067 mode=indexing
              shift-right: [w1073] -> w1060
              shift-left: w1059 -> [_]
              shift-right: [w1072] -> w1057
              shift-left: w1058 -> [_]
              i -> [w1079]
              n523 = call-dynamic "get waveform - 8bit.vi"("Waveform Obj 입력"=w1081) -> ("8bit memory data"=w1071:u8[], "Waveform Obj 출력"=w1074:refnum<class "Waveform Obj.lvclass">)  [unwired: 7 in, 2 out]
              n524 = property class="Waveform Obj.lvclass"(reference=w1074) -> ("Accessors:voltage range"=w1073:dbl, "Accessors:wait"=w1072:u8, "Accessors:name"=w1080:string)  [unwired: 1 in, 2 out]
              n525 = Array Size(array=w1071) -> (size(s)=w1070:i32)
              n526 = Number To Decimal String(number=w1070) -> (decimal integer string=w1075:string)  [unwired: 1 in]
              n527 = Increment(x=w1079) -> (x+1=w1076:i32)
              n528 = Number To Decimal String(number=w1076) -> (decimal integer string=w1078:string)  [unwired: 1 in]
              n529 = Build Array(w1080, w1075) -> (w1077:string[])
            }
            n530 = Add Array Elements(numeric array=w1067) -> (sum=→"WF Seq_Total Bytes":i32)
            n531 = Empty Array?(array=w1063) -> (empty?=w1062:bool)
            n532 = property on="WF Seq" class="MCListbox (엄격한)"("RowHdrs[]"=w1063, "ItemNames"=w1068) -> ()  [unwired: 2 in, 2 out]
            n533 = local write "WF Seq_Voltage Range"(w1060) -> ()
            n534 = local write "WF Seq_Wait"(w1057) -> ()
            n535 = Select(t=T17."Disabled and Grayed Out" ("비활성화"), s=w1062, f=T17."Enabled" ("비활성화")) -> (s? t:f=w1061:T17)
            n536 = property on="WF Seq_View" class="Bool"("DisabledEnum"=w1061) -> ()  [unwired: 2 in, 2 out]
            n537 = property on="WF Seq_Up" class="Bool"("DisabledEnum"=w1061) -> ()  [unwired: 2 in, 2 out]
            n538 = property on="WF Seq_Down" class="Bool"("DisabledEnum"=w1061) -> ()  [unwired: 2 in, 2 out]
            n539 = property on="WF Seq_Rename" class="Bool"("DisabledEnum"=w1061) -> ()  [unwired: 2 in, 2 out]
            n540 = property on="WF Seq_Delete" class="Bool"("DisabledEnum"=w1061) -> ()  [unwired: 2 in, 2 out]
            n541 = property on="WF Seq_Save File" class="Bool"("DisabledEnum"=w1061) -> ()  [unwired: 2 in, 2 out]
            n542 = property on="WF Seq_Add to List" class="Bool"("DisabledEnum"=w1061) -> ()  [unwired: 2 in, 2 out]
          }
          frame "WF List" {
            n543 = local read "WF List_Sampling Rate"() -> (w1086:u32)
            n544 = for {
              tunnel: [w1105] -> w1097 mode=indexing
              tunnel: [w1106] -> w1094 mode=indexing
              tunnel: w1088 -> [w1103] mode=indexing
              tunnel: [w1098] -> w1085 mode=indexing
              tunnel: w1086 -> [w1099]
              i -> [w1107]
              n545 = Unbundle By Name(w1103) -> ("Name"=w1100:string, "WF Seq"=w1101:refnum<class "Waveform Obj.lvclass">[])
              n546 = call "(SubVI)Waveform Editor_Build WF Seq.vi"("Name (empty)"=w1100, "Sampling Rate"=w1099, "WF Seq"=w1101) -> ("bytes of memory data"=w1098:i32)  [unwired: 3 in, 5 out]
              n547 = Number To Decimal String(number=w1098) -> (decimal integer string=w1102:string)  [unwired: 1 in]
              n548 = Increment(x=w1107) -> (x+1=w1104:i32)
              n549 = Number To Decimal String(number=w1104) -> (decimal integer string=w1106:string)  [unwired: 1 in]
              n550 = Build Array(w1100, w1102) -> (w1105:string[])
            }
            n551 = Add Array Elements(numeric array=w1085) -> (sum=→"WF List_Total Bytes":i32)
            n552 = global read "(Var)System Variables.vi" "Haptic IC"() -> (w1084:refnum<class "Haptic IC.lvclass">)
            n553 = Empty Array?(array=w1094) -> (empty?=w1093:bool)
            n554 = property on="WF List" class="MCListbox (엄격한)"("RowHdrs[]"=w1094, "ItemNames"=w1097) -> (error out=w1092:errorcluster)  [unwired: 2 in, 1 out]
            n555 = property on="WF List" class="MCListbox (엄격한)"(error in=w1092) -> (error out=w1090:errorcluster, "Value"=w1091:i32[])  [unwired: 1 in, 1 out]
            n556 = call-dynamic "check memory limit.vi"("bytes of waveform"=w1085, "Haptic IC 입력"=w1084) -> ("message"=w1082:string, "disable?"=w1083:T17)  [unwired: 6 in, 2 out]
            n557 = property on="WF List_Mem Update" class="Bool"("DisabledEnum"=w1083, "TipStrip"=w1082) -> ()  [unwired: 2 in, 2 out]
            n558 = property on="WF List" class="MCListbox (엄격한)"(error in=w1090, "Val(Sgnl)"=w1091) -> ()  [unwired: 1 in, 2 out]
            n559 = Select(t=T17."Disabled and Grayed Out" ("비활성화"), s=w1093, f=T17."Enabled" ("비활성화")) -> (s? t:f=w1089:T17)
            n560 = property on="WF List_View" class="Bool"("DisabledEnum"=w1089) -> ()  [unwired: 2 in, 2 out]
            n561 = property on="WF List_Up" class="Bool"("DisabledEnum"=w1089) -> ()  [unwired: 2 in, 2 out]
            n562 = property on="WF List_Down" class="Bool"("DisabledEnum"=w1089) -> ()  [unwired: 2 in, 2 out]
            n563 = property on="WF List_Rename" class="Bool"("DisabledEnum"=w1089) -> ()  [unwired: 2 in, 2 out]
            n564 = property on="WF List_Delete" class="Bool"("DisabledEnum"=w1089) -> ()  [unwired: 2 in, 2 out]
            n565 = property on="WF List_Save File" class="Bool"("DisabledEnum"=w1089) -> ()  [unwired: 2 in, 2 out]
            n566 = property on="WF List_Export" class="Bool"("DisabledEnum"=w1089) -> ()  [unwired: 2 in, 2 out]
          }
        }
      }
      event "Graph": Cursor Move {
        n567 = event-data() -> ("CursLoc"=w1111:cluster{"X":dbl, "Y":dbl})  [unwired: 1 in, 8 out]
        n568 = Unbundle By Name(w1111) -> ("X"=→"Graph_Cursor X":dbl, "Y"=→"Graph_Cursor Y":dbl)
      }
      event User Event {
        # "Vibration Scope에서 \nScope Start 시 RTP Start, Memory Update 비활성화\nScope Stop 시 RTP Start, Memory Update를 조건에 따라 활성화 하도록 이벤트 발생"
        n569 = event-data() -> ("Mode Event"=w1115:T20)  [unwired: 1 in, 4 out]
        n570 = case shown="\"RTP Play\", 기본" w1115 {
          tunnel: w1114 -> [_ _ w1121]
          frame "RTP Play", Default {
          }
          frame "Scope Start" {
            w1119 = T17."Disabled and Grayed Out" ("비활성화")
            n571 = property on="WF List_RTP Start" class="Bool"("DisabledEnum"=w1119) -> ()  [unwired: 2 in, 2 out]
            n572 = property on="WF List_Mem Update" class="Bool"("DisabledEnum"=w1119) -> ()  [unwired: 2 in, 2 out]
          }
          frame "Scope Stop" {
            n573 = local read "WF List"() -> (w1122:i32[])
            n574 = property on="WF List" class="MCListbox (엄격한)"("Val(Sgnl)"=w1122) -> ()  [unwired: 2 in, 2 out]
            n575 = Generate User Event(user event=w1121, event data cluster=(Ctrl)Waveform_Editor_Update_Listbox_User_Event."WF List" ("이벤트 데이터")) -> ()  [unwired: 2 in, 2 out]
          }
        }
      }
    }
  }
  n576 = disable-structure shown="비활성화" {
    frame Disabled {
      n577 = Generate User Event(event data cluster=(Ctrl)Waveform_Editor_Update_Graph_User_Event."WF List" ("이벤트 데이터")) -> ()  [unwired: 3 in, 2 out]
      n578 = Generate User Event(event data cluster=(Ctrl)Waveform_Editor_Update_Listbox_User_Event."WF List" ("이벤트 데이터")) -> ()  [unwired: 3 in, 2 out]
    }
    frame Enabled {
    }
  }
  n579 = Unregister For Events(event registration refnum=w29) -> ()  [unwired: 1 in, 1 out]
  n580 = Release Queue(queue=w16, error in (no error)=w15) -> ()  [unwired: 1 in, 3 out]
  n581 = case shown="참" w3 {
    frame False {
    }
    frame True {
      n582 = invoke class="VI" method="FP.Close"() -> ()  [unwired: 3 in, 3 out]
    }
  }
